vi "Live Capture Functional Stack.10.64bit.vi"() -> ()   [LabVIEW 2014]
uses:
  subvis/Stack Track.ctl
  subvis/Stack_State.ctl
  CameraControlTypeDef.ctl
  Desktop/camtiff/ctiff.llb/__CTIFFNewFileAndStyleUINT16.vi
  Desktop/camtiff/ctiff.llb/__CTIFFAddNewPageUINT16.vi
panel:
  in  "Preview":bool
  in  "Capture Mode":bool
  out "Record Ready":bool
  in  "Stacks":dbl=1.0
  out "Stack Frames":i32=100
  in  "Stack Frames":i32=100
  in  "Temp":path=path "C:/temp.tmp"
  in  "Frames":i32=100
  in  "HardDisk Record":bool
  in  "Internal Line Interval":dbl
  in  "Slit Width / Lines":sgl=150.0
  in  "Camera Readout Mode":u16(ring)=12 items=["Full Frame"=1, "Slit Scanning"=12]
  in  "Readout Direction":sgl(ring)=1.0 items=["Forward"=1, "Backward"=2]
  in  "Trigger Mode":sgl(ring)=1.0 items=["Normal"=1, "Start "=6]
  in  "Trigger Source":sgl(ring)=2.0 items=["Internal"=1, "External"=2]
  out "State":T1=enum."Start Sequence"
  out "Image":u16[][](graph)
  out "Saving":bool
  in  "AutoIncrement":bool=TRUE
  in  "Path":path=path "C:/Users/spim/Desktop/Craig Cap/temp/a.tiff"
  in  "Frames":i32=100
  out "Frame Index":i32
  out "error out":errorcluster
  in  "stop":bool
  in  "Ram Record":bool
  out "Total Frames":i32
  out "Elapsed Time":u32
  out "Software FPS":dbl
  out "Camera FPS":dbl
  in  "H Offset":i32 min=0 max=0 step=4
  in  "H Width":i32 min=4 max=2048 step=4
  out "SMD":dbl
  out "SHO":i32
  in  "V Offset":i32 min=0 max=0 step=4
  in  "V Width":i32 min=4 max=2048 step=4
  in  "Binning":u16(ring) items=["1x1"=1, "2x2"=2, "4x4"=4]
  out "SHW":i32
  out "SVO":i32
  out "SVW":i32
  in  "Scan Mode":dbl min=1.0 max=2.0 step=1.0
  in  "Exposure":dbl min=0.0010036691729323308 max=10.000004210526315 step=1e-08
  out "EXP":dbl
  out "Camera Model":string
  out "Camera Version":string
  out "Camera Serial":string
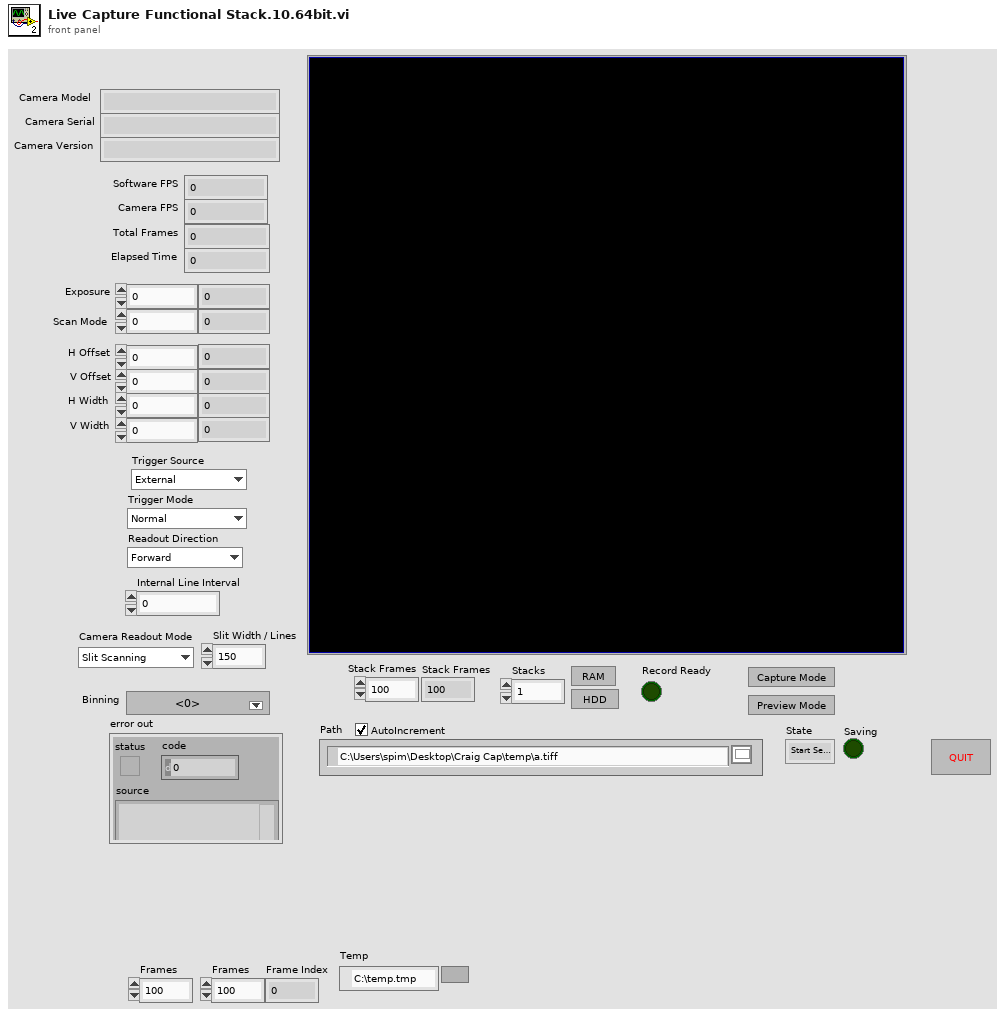
[diagram p1: front panel]
types:
  T1 = typedef "Stack Track.ctl" = enum16{"Idle", "Start Sequence", "Read Disk", "STOP", "Collecting", "End"}
  T2 = typedef "CameraControlTypeDef.ctl" = enum16{"IntervalLineInt", "Ram Record", "HardDisk Record", "Disengage Update", "Update", "Idle", "ROI", "Binning", "Scan Mode", "Trigger Mode", "Readout Mode", "Readout Direction", "Preview"}
  T3 = typedef "Stack_State.ctl" = cluster{"State":T1, "Stack Number":i32, "Image":u16[][], "Stacks":i32}
  T4 = enum8{"Enabled", "Disabled", "Disabled and Grayed Out"}
  T5 = cluster{"Model":string, "Camera ID":string, "Firmware":string}
  T6 = cluster{"Value":i32, "Minimum":i32, "Maximum":i32, "Increment":i32}
  T7 = cluster{"height":u32, "width":u32, "datatype":u32}
  T8 = cluster{"H Offset":i32, "V Offset":i32, "H Width":i32, "V Width":i32}
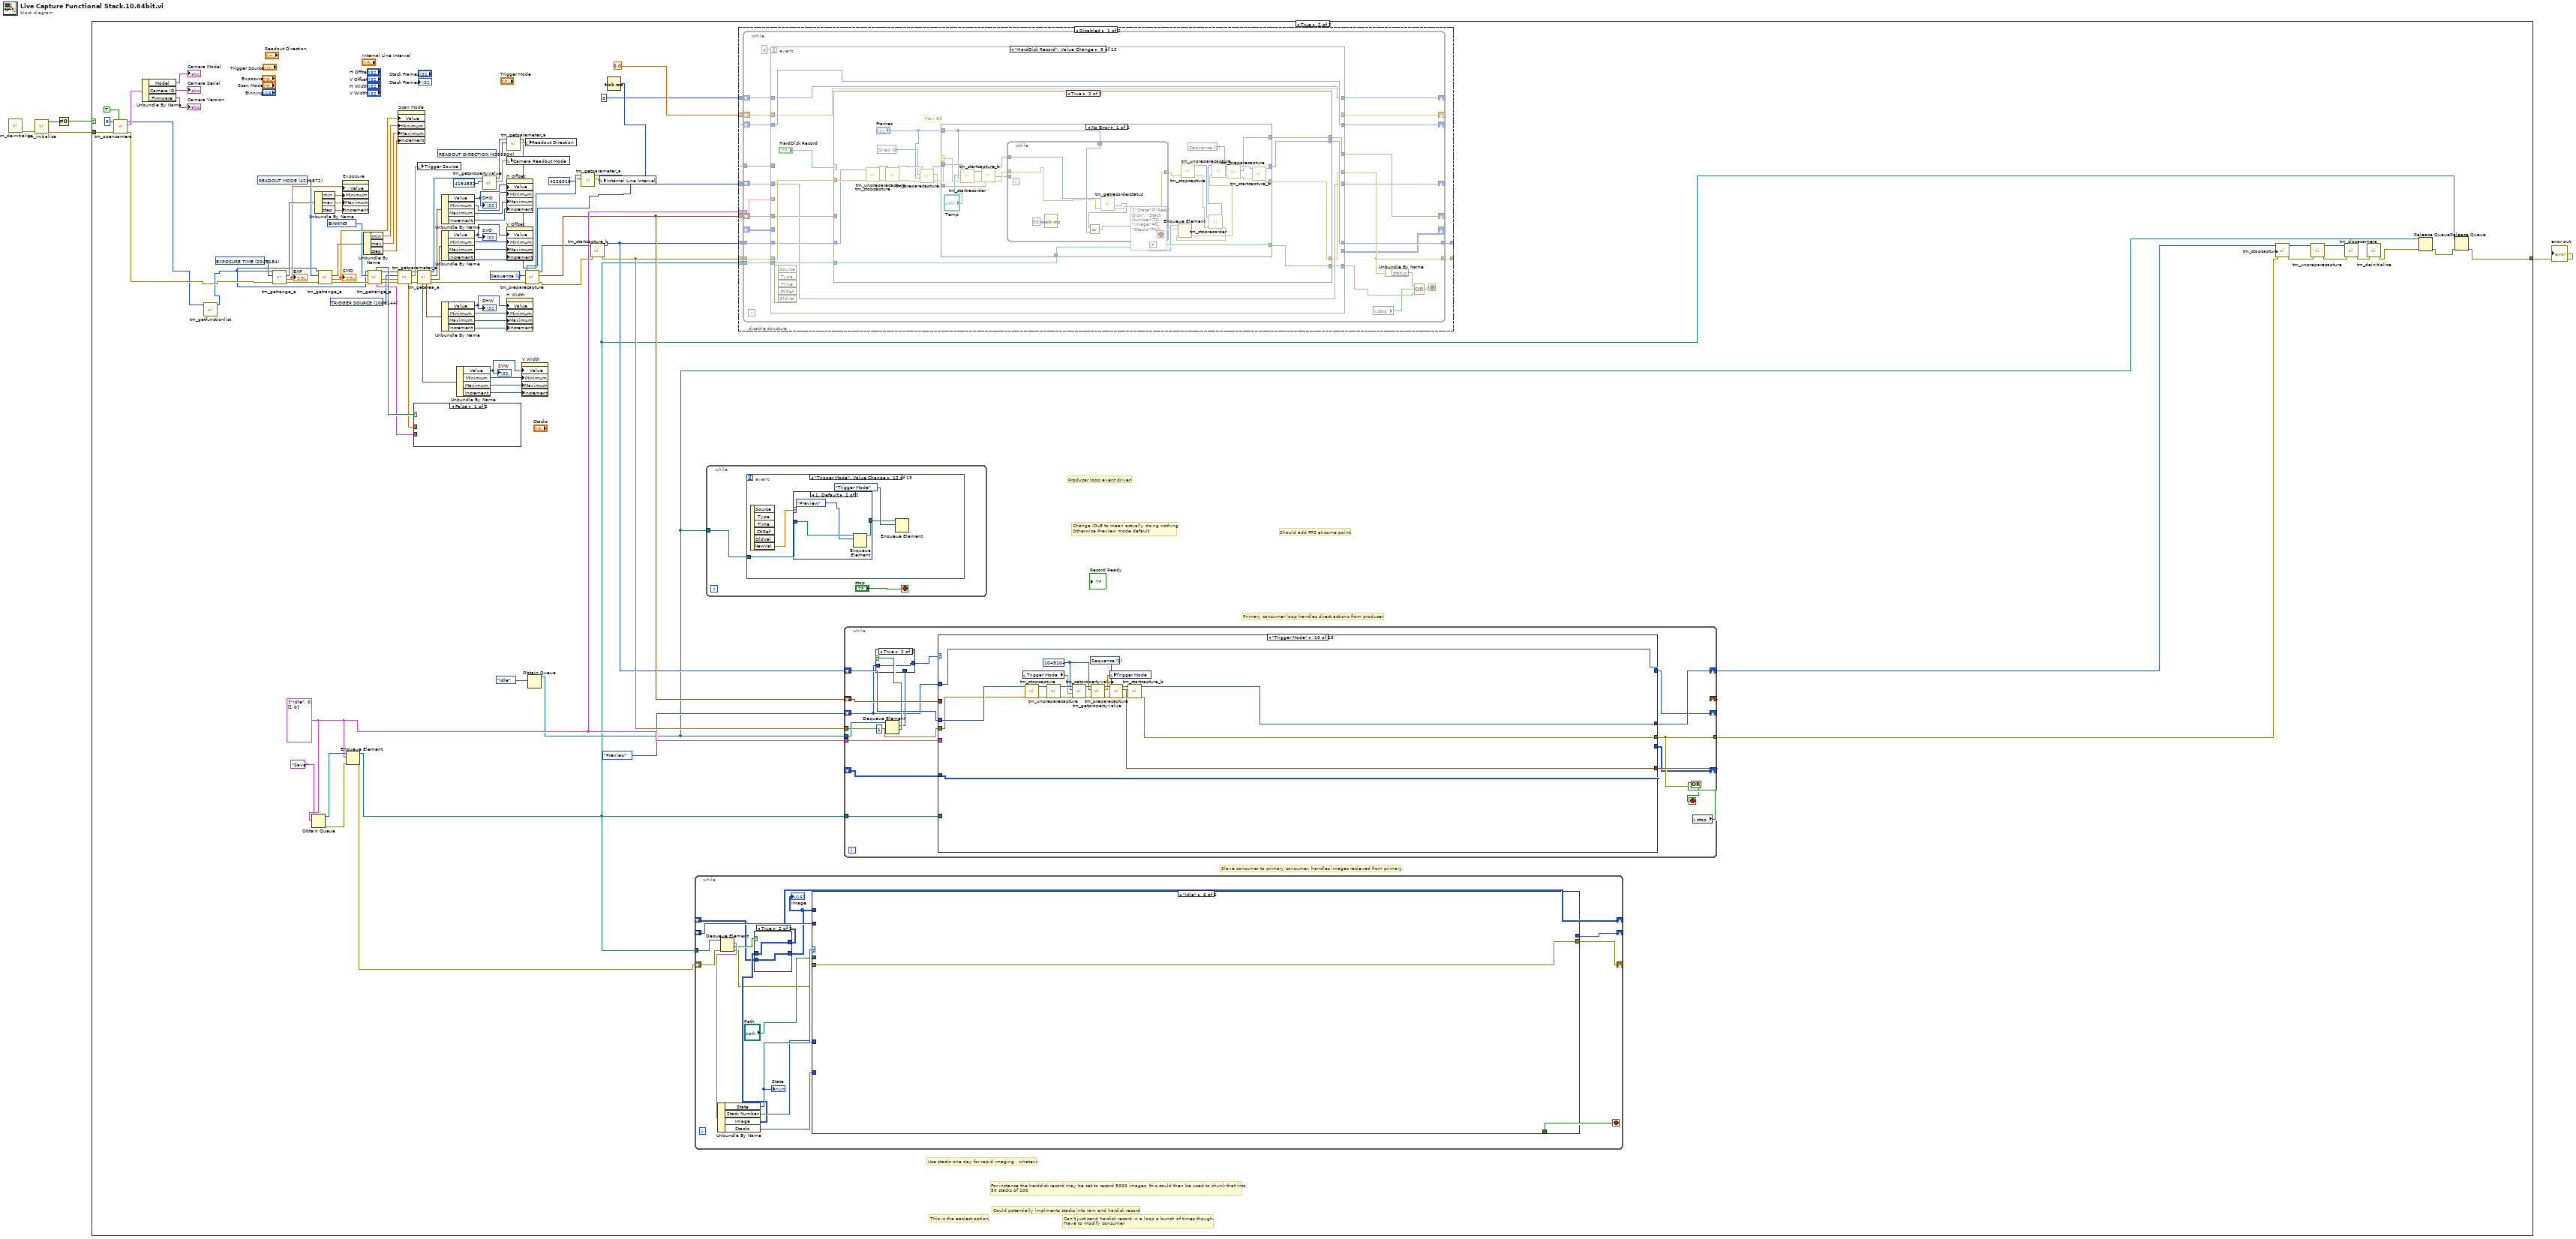
[diagram p0: block diagram]
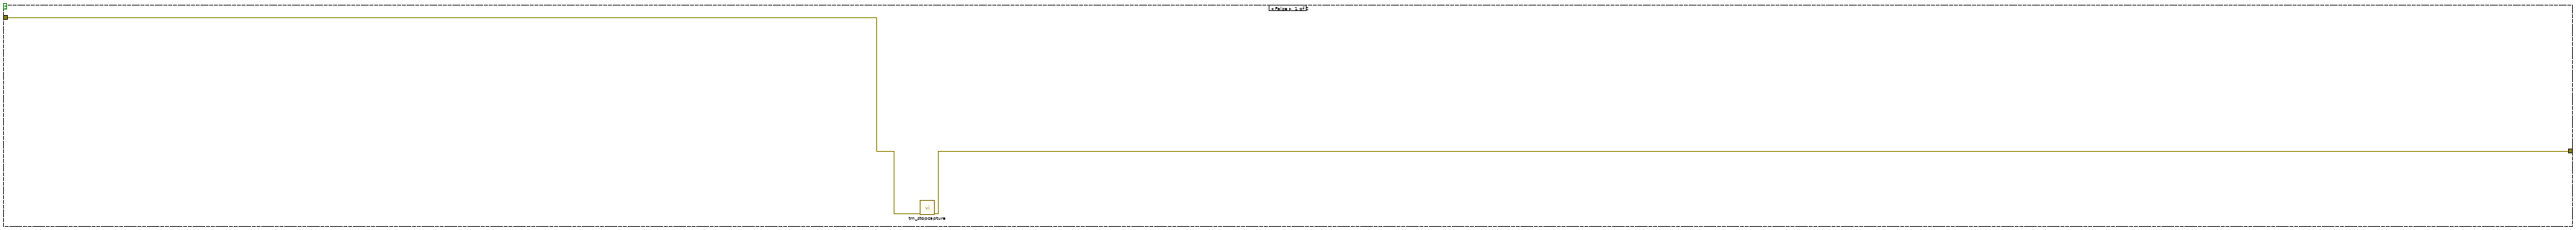
[diagram p2: hidden frame]
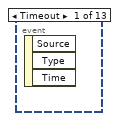
[diagram p3: hidden frame]
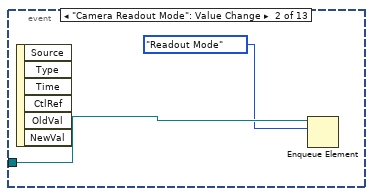
[diagram p4: hidden frame]
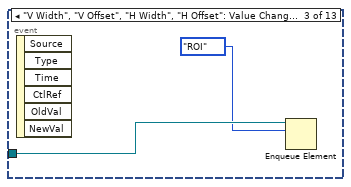
[diagram p5: hidden frame]
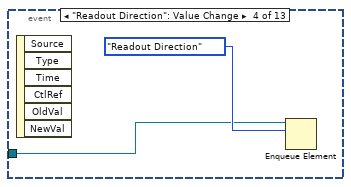
[diagram p6: hidden frame]
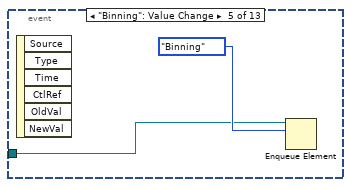
[diagram p7: hidden frame]
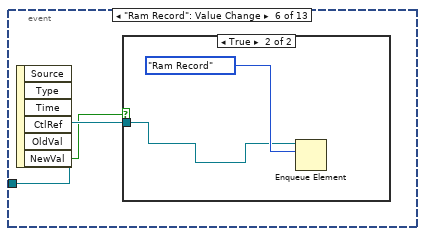
[diagram p8: hidden frame]
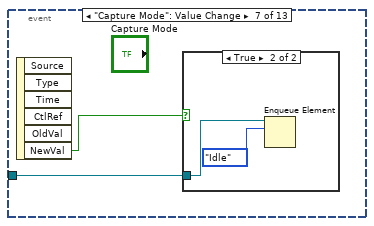
[diagram p10: hidden frame]
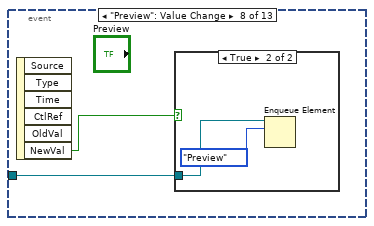
[diagram p12: hidden frame]
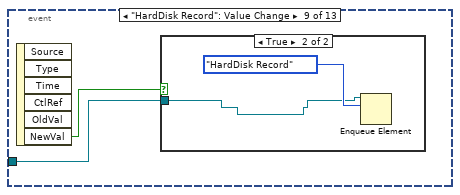
[diagram p14: hidden frame]
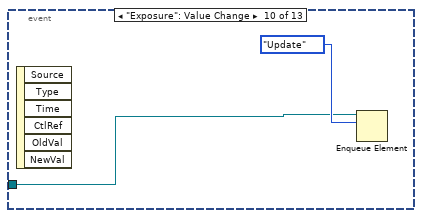
[diagram p16: hidden frame]
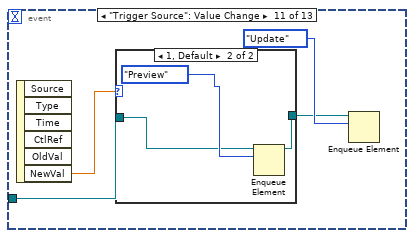
[diagram p17: hidden frame]
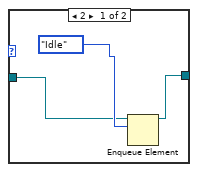
[diagram p18: hidden frame]
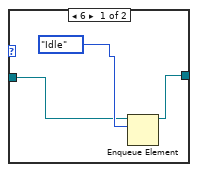
[diagram p19: hidden frame]
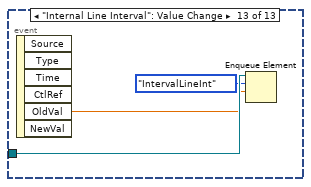
[diagram p20: hidden frame]
diagram:
  n1 = call <userlib>:"tm_deinitialize.vi"() -> ("error out"=w1:errorcluster)  [unwired: 11 in]
  n2 = call <userlib>:"tm_initialize.vi"("error in (no error)"=w1) -> ("error out"=w3:errorcluster, "Number Of Cameras"=w2:u32)  [unwired: 7 in, 2 out]
  n3 = Not Equal To 0?(x=w2) -> (x != 0?=w5:bool)
  n4 = case shown="True" w5 {
    tunnel: [w6 w17] -> w4
    tunnel: w3 -> [w7 w100]
    frame False {
      n5 = call <userlib>:"tm_stopcapture.vi"("error in (no error)"=w7) -> ("error out"=w6:errorcluster)  [unwired: 9 in, 1 out]
    }
    frame True {
      w35 = u32 4211904 items=["SENSOR MODE"=4212128, "CCD MODE"=4212384, "READOUT MODE"=4211872, "ACTIVE VIEW INDEX"=4343136, "BITS PER CHANNEL"=4342976, "IMAGE PIXEL TYPE"=4343296, "BINNING"=4215968, "EXPOSURE TIME"=2049184, "CONTRAST GAIN"=3163312, "CONTRAST OFFSET"=3163328, "LIGHT MODE"=2114720, "SENSITIVITY"=2114992, "PHOTON IMAGING MODE"=2115200, "HIGH DYNAMIC RANGE MODE"=3163360, "WHITE BALANCE"=3163568, "TEMPERATURE"=2115232, "TEMPERATURE TARGET"=2115264, "SENSOR COOLER FAN"=2115296, "LINEBUNDLE HEIGHT"=4212192, "MECHANICAL SHUTTER"=2115488, "BACK FOCUS POSITION"=8422304, "TRIGGER CONNECTOR"=1066432, "TRIGGER SOURCE"=1066144, "OUTPUT TRIGGER SOURCE"=1852576, "TRIGGER GLOBAL EXPOSURE"=2049680, "FIRST TRIGGER BEHAVIOR"=2049696, "CHANNEL SYNC"=1852352, "READOUT DIRECTION"=4211904, "PRE HSYNC COUNT"=1852704] ("Parameter")
      w44 = u32 1066144 items=["SENSOR MODE"=4212128, "CCD MODE"=4212384, "READOUT MODE"=4211872, "ACTIVE VIEW INDEX"=4343136, "BITS PER CHANNEL"=4342976, "IMAGE PIXEL TYPE"=4343296, "BINNING"=4215968, "EXPOSURE TIME"=2049184, "CONTRAST GAIN"=3163312, "CONTRAST OFFSET"=3163328, "LIGHT MODE"=2114720, "SENSITIVITY"=2114992, "PHOTON IMAGING MODE"=2115200, "HIGH DYNAMIC RANGE MODE"=3163360, "WHITE BALANCE"=3163568, "TEMPERATURE"=2115232, "TEMPERATURE TARGET"=2115264, "SENSOR COOLER FAN"=2115296, "LINEBUNDLE HEIGHT"=4212192, "MECHANICAL SHUTTER"=2115488, "BACK FOCUS POSITION"=8422304, "TRIGGER CONNECTOR"=1066432, "TRIGGER SOURCE"=1066144, "OUTPUT TRIGGER SOURCE"=1852576, "TRIGGER GLOBAL EXPOSURE"=2049680, "FIRST TRIGGER BEHAVIOR"=2049696, "CHANNEL SYNC"=1852352, "READOUT DIRECTION"=4211904, "PRE HSYNC COUNT"=1852704] ("Parameter")
      w30 = T3 {"State"=enum."Idle", "Stack Number"=0, "Image"=[], "Stacks"=0} ("input cluster")
      w49 = u32 2049184 items=["BINNING"=4215968, "BITS PER CHANNEL"=4342976, "ACTIVE VIEW INDEX"=4343136, "CCD MODE"=4212384, "SENSOR MODE"=4212128, "READOUT MODE"=4211872, "EXPOSURE TIME"=2049184, "CONTRAST GAIN"=3163312, "CONTRAST OFFSET"=3163328, "LIGHT MODE"=2114720, "SENSITIVITY"=2114992, "WHITE BALANCE"=3163568, "PHOTON IMAGING MODE"=2115200, "HIGH DYNAMIC RANGE MODE"=3163360, "TRIGGER SOURCE"=1066144, "TRIGGER ACTIVE"=1066160, "TRIGGER MODE"=1066400, "TRIGGER POLARITY"=1066416, "TRIGGER GLOBAL EXPOSURE"=2049680, "FIRST TRIGGER BEHAVIOR"=2049696, "TRIGGER TIMES"=1066448, "OUTPUT TRIGGER POLARITY"=1852592, "OUTPUT TRIGGER DELAY"=1852624, "OUTPUT TRIGGER PERIOD"=1852640, "TEMPERATURE"=2115232, "TEMPERATURE TARGET"=2115264, "SENSOR COOLER FAN"=2115296, "MECHANICAL SHUTTER"=2115488, "BACK FOCUS POSITION"=8422304, "FRAMEBUNDLE MODE"=4346784, "FRAMEBUNDLE NUMBER"=4346800, "LINEBUNDLE HEIGHT"=4212192, "TRIGGER CONNECTOR"=1066432, "IMAGE PIXEL TYPE"=4343296, "OUTPUT TRIGGER KIND"=1852656, "READOUT DIRECTION"=4211904, "CHANNEL SYNC"=1852352] ("Parameter")
      w50 = u32 4211872 items=["BINNING"=4215968, "BITS PER CHANNEL"=4342976, "ACTIVE VIEW INDEX"=4343136, "CCD MODE"=4212384, "SENSOR MODE"=4212128, "READOUT MODE"=4211872, "EXPOSURE TIME"=2049184, "CONTRAST GAIN"=3163312, "CONTRAST OFFSET"=3163328, "LIGHT MODE"=2114720, "SENSITIVITY"=2114992, "WHITE BALANCE"=3163568, "PHOTON IMAGING MODE"=2115200, "HIGH DYNAMIC RANGE MODE"=3163360, "TRIGGER SOURCE"=1066144, "TRIGGER ACTIVE"=1066160, "TRIGGER MODE"=1066400, "TRIGGER POLARITY"=1066416, "TRIGGER GLOBAL EXPOSURE"=2049680, "FIRST TRIGGER BEHAVIOR"=2049696, "TRIGGER TIMES"=1066448, "OUTPUT TRIGGER POLARITY"=1852592, "OUTPUT TRIGGER DELAY"=1852624, "OUTPUT TRIGGER PERIOD"=1852640, "TEMPERATURE"=2115232, "TEMPERATURE TARGET"=2115264, "SENSOR COOLER FAN"=2115296, "MECHANICAL SHUTTER"=2115488, "BACK FOCUS POSITION"=8422304, "FRAMEBUNDLE MODE"=4346784, "FRAMEBUNDLE NUMBER"=4346800, "LINEBUNDLE HEIGHT"=4212192, "TRIGGER CONNECTOR"=1066432, "IMAGE PIXEL TYPE"=4343296, "OUTPUT TRIGGER KIND"=1852656, "READOUT DIRECTION"=4211904, "CHANNEL SYNC"=1852352] ("Parameter")
      w51 = u32 4215968 items=["BINNING"=4215968, "BITS PER CHANNEL"=4342976, "ACTIVE VIEW INDEX"=4343136, "CCD MODE"=4212384, "SENSOR MODE"=4212128, "READOUT MODE"=4211872, "EXPOSURE TIME"=2049184, "CONTRAST GAIN"=3163312, "CONTRAST OFFSET"=3163328, "LIGHT MODE"=2114720, "SENSITIVITY"=2114992, "WHITE BALANCE"=3163568, "PHOTON IMAGING MODE"=2115200, "HIGH DYNAMIC RANGE MODE"=3163360, "TRIGGER SOURCE"=1066144, "TRIGGER ACTIVE"=1066160, "TRIGGER MODE"=1066400, "TRIGGER POLARITY"=1066416, "TRIGGER GLOBAL EXPOSURE"=2049680, "FIRST TRIGGER BEHAVIOR"=2049696, "TRIGGER TIMES"=1066448, "OUTPUT TRIGGER POLARITY"=1852592, "OUTPUT TRIGGER DELAY"=1852624, "OUTPUT TRIGGER PERIOD"=1852640, "TEMPERATURE"=2115232, "TEMPERATURE TARGET"=2115264, "SENSOR COOLER FAN"=2115296, "MECHANICAL SHUTTER"=2115488, "BACK FOCUS POSITION"=8422304, "FRAMEBUNDLE MODE"=4346784, "FRAMEBUNDLE NUMBER"=4346800, "LINEBUNDLE HEIGHT"=4212192, "TRIGGER CONNECTOR"=1066432, "IMAGE PIXEL TYPE"=4343296, "OUTPUT TRIGGER KIND"=1852656, "READOUT DIRECTION"=4211904, "CHANNEL SYNC"=1852352] ("Parameter")
      w96 = 1 items=["Snap", "Sequence"] ("Capture mode")
      # "Can't just send hardisk record in a loop a bunch of times though.\nHave to modify consumer"
      # "This is the easiest option."
      # "Could potentially implments stacks into ram and hardisk record"
      # "For instance the harddisk record may be set to record 5000 images, this could then be used to chunk that into\n50 stacks of 100"
      # "Use stacks one day for rapid imaging , whatevr."
      # "Change IDLE to mean actually doing nothing\nOtherwise Preview mode default"
      # "Slave consumer to primary consumer, handles images recieved from primary."
      # "Primary consumer loop handles direct actions from producer"
      # "Producer loop event driven"
      # "Should add FPS at some point."
      n6 = call <userlib>:"tm_opencamera.vi"("Force Open"=TRUE, "error in (no error)"=w100, "Camera Index"=u32 0) -> ("error out"=w31:errorcluster, "Camera Details"=w63:T5, "Handle out"=w15:u32)  [unwired: 6 in]
      n7 = Unbundle By Name(w63) -> ("Model"=→"Camera Model":string, "Camera ID"=→"Camera Serial":string, "Firmware"=→"Camera Version":string)
      n8 = call <userlib>:"tm_getfunctionlist.vi"("Handle in"=w15) -> ("Handle out"=w14:u32)  [unwired: 8 in, 2 out]
      n9 = call <userlib>:"tm_getrange_a.vi"("error in (no error)"=w31, "Parameter"=w49, "Handle in"=w14) -> ("error out"=w58:errorcluster, "default"=w47:dbl, "Range"=w59:cluster{"min":dbl, "max":dbl, "step":dbl})  [unwired: 2 in, 4 out]
      "EXP" <- w47
      n10 = Obtain Queue(name (unnamed)="Save", element data type=w30) -> (queue out=w33:refnum<queue>, error out=w12:errorcluster)  [unwired: 3 in, 1 out]
      n11 = Unbundle By Name(w59) -> ("min"=w94:dbl, "max"=w93:dbl, "step"=w92:dbl)
      n12 = call <userlib>:"tm_getrange_a.vi"("error in (no error)"=w58, "Parameter"=w50, "Handle in"=w14) -> ("error out"=w55:errorcluster, "default"=w56:dbl, "Range"=w57:cluster{"min":dbl, "max":dbl, "step":dbl})  [unwired: 2 in, 4 out]
      "SMD" <- w56
      n13 = property on="Exposure" class="DigNum (strict)"("Value"=w47, "Minimum"=w94, "Maximum"=w93, "Increment"=w92) -> ()  [unwired: 2 in, 2 out]
      n14 = Enqueue Element(queue=w33, element=w30, error in (no error)=w12) -> (queue out=w16:refnum<queue>, error out=w11:errorcluster)  [unwired: 1 in, 1 out]
      n15 = Unbundle By Name(w57) -> ("min"=w91:dbl, "max"=w90:dbl, "step"=w89:dbl)
      n16 = call <userlib>:"tm_getrange_a.vi"("error in (no error)"=w55, "Parameter"=w51, "Handle in"=w14) -> ("error out"=w41:errorcluster, "default"=w53:dbl, "Handle out"=w43:u32, "Value Names"=w52:cluster{"Name":string, "Value":dbl}[], "Writable"=w54:bool)  [unwired: 2 in, 2 out]
      n17 = property on="Scan Mode" class="DigNum (strict)"("Value"=w56, "Minimum"=w91, "Maximum"=w90, "Increment"=w89) -> ()  [unwired: 2 in, 2 out]
      n18 = call <userlib>:"tm_getparameter_a.vi"("error in (no error)"=w41, "Parameter"=w44, "Handle in"=w43) -> ("error out"=w40:errorcluster, "Value out"=w45:dbl, "Handle out"=w42:u32)  [unwired: 6 in]
      n19 = case shown="False" w54 {
        tunnel: w52 -> [_ w1193]
        tunnel: w53 -> [_ w1192]
        frame False {
        }
        frame True {
          n20 = property on="Binning" class="Ring (strict)"("Value"=w1192, "StringsAndValues[]"=w1193) -> ()  [unwired: 2 in, 2 out]
        }
      }
      n21 = local write "Trigger Source"(w45) -> ()
      n22 = call <userlib>:"tm_getarea_a.vi"("error in (no error)"=w40, "Handle in"=w42) -> ("error out"=w46:errorcluster, "V Offset"=w88:T6, "H Offset"=w69:T6, "Handle out"=w37:u32, "H Width"=w87:T6, "V Width"=w86:T6)  [unwired: 4 in]
      n23 = Unbundle By Name(w69) -> ("Value"=w68:i32, "Minimum"=w67:i32, "Maximum"=w66:i32, "Increment"=w65:i32)
      "SHO" <- w68
      n24 = Unbundle By Name(w88) -> ("Value"=w76:i32, "Minimum"=w85:i32, "Maximum"=w84:i32, "Increment"=w83:i32)
      "SVO" <- w76
      n25 = Unbundle By Name(w87) -> ("Value"=w75:i32, "Minimum"=w82:i32, "Maximum"=w81:i32, "Increment"=w80:i32)
      "SHW" <- w75
      n26 = Unbundle By Name(w86) -> ("Value"=w74:i32, "Minimum"=w79:i32, "Maximum"=w78:i32, "Increment"=w77:i32)
      "SVW" <- w74
      n27 = call <userlib>:"tm_getpropertyvalue.vi"("Property ID"=u32 4194832, "Handle in"=w37) -> ("Value in"=w38:sgl, "Handle out"=w36:u32)  [unwired: 7 in, 1 out]
      n28 = call <userlib>:"tm_getparameter_a.vi"("Parameter"=w35, "Handle in"=w36) -> ("Value out"=w34:dbl, "Handle out"=w21:u32)  [unwired: 7 in, 1 out]
      n29 = local write "Camera Readout Mode"(w38) -> ()
      n30 = property on="H Offset" class="DigNum (strict)"("Value"=w68, "Minimum"=w67, "Maximum"=w66, "Increment"=w65) -> ()  [unwired: 2 in, 2 out]
      n31 = property on="V Offset" class="DigNum (strict)"("Value"=w76, "Minimum"=w85, "Maximum"=w84, "Increment"=w83) -> ()  [unwired: 2 in, 2 out]
      n32 = property on="H Width" class="DigNum (strict)"("Value"=w75, "Minimum"=w82, "Maximum"=w81, "Increment"=w80) -> ()  [unwired: 2 in, 2 out]
      n33 = property on="V Width" class="DigNum (strict)"("Value"=w74, "Minimum"=w79, "Maximum"=w78, "Increment"=w77) -> ()  [unwired: 2 in, 2 out]
      n34 = local write "Readout Direction"(w34) -> ()
      n35 = Obtain Queue(element data type=CameraControlTypeDef."Idle" ("Enum")) -> (queue out=w19:refnum<queue>)  [unwired: 4 in, 2 out]
      n36 = call <userlib>:"tm_getparameter_a.vi"("Parameter"=4226016, "Handle in"=w21) -> ("Value out"=w9:dbl, "Handle out"=w10:u32)  [unwired: 7 in, 1 out]
      n37 = call <userlib>:"tm_preparecapture.vi"("error in (no error)"=w46, "Capture mode"=w96, "Handle in"=w10) -> ("error out"=w32:errorcluster, "Buffer Info"=w29:T7, "Handle out"=w22:u32)  [unwired: 5 in, 1 out]
      n38 = call <userlib>:"tm_startcapture_b.vi"("error in (no error)"=w32, "Handle in"=w22) -> ("error out"=w27:errorcluster, "Handle out"=w28:u32)  [unwired: 8 in]
      n39 = local write "Internal Line Interval"(w9) -> ()
      n40 = Tick Count (ms)() -> (millisecond timer value=w95:u32)
      n41 = while {
        tunnel: w16 -> [w1109]
        shift-right: [w1105] -> _
        shift-left: _ -> [w1103]
        shift-right: [w1102] -> _
        shift-left: w11 -> [w1095]
        shift-right: [w1100] -> _
        shift-left: _ -> [w1096]
        stop <- w1104 stop-if-true
        n42 = Dequeue Element(queue=w1109, error in (no error)=w1095) -> (element=w1108:T3, timed out?=w1097:bool, error out=w1094:errorcluster)  [unwired: 1 in, 1 out]
        n43 = Unbundle By Name(w1108) -> ("State"=w1107:T1, "Stack Number"=w1106:i32, "Image"=w1098:u16[][], "Stacks"=w1093:i32)
        "State" <- w1107
        n44 = case shown="True" w1097 {
          tunnel: w1098 -> [w1111 w1113]
          tunnel: [w1111 w1112] -> w1099
          tunnel: [w1110 w1113] -> w1100
          tunnel: w1096 -> [w1110 w1112]
          frame False {
          }
          frame True {
          }
        }
        "Image" <- w1099
        n45 = case shown="\"Idle\"" w1107 {
          tunnel: w1106 -> [_ _ _ _ _ _]
          tunnel: [w1116 w1133 _ _ _ _] -> w1105
          tunnel: w1103 -> [_ w1134 w1140 _ _ _]
          tunnel: [FALSE _ _ _ TRUE _] -> w1104
          tunnel: w1099 -> [w1114 w1135 _ _ _ _]
          tunnel: w1094 -> [_ w1132 w1138 w1153 w1189 w1191]
          tunnel: [w1117 w1131 w1139 w1150 w1189 w1191] -> w1102
          tunnel: "Path" -> [w1120 _ _ w1143 _ _]
          tunnel: w1093 -> [_ _ _ w1146 _ _]
          frame "Start Sequence" {
            # "Public tiff library"
            # "Get path and open file"
            n46 = Equal?(x=w1120, y=path "") -> (x = y?=w1122:bool)
            n47 = case shown="True" w1122 {
              tunnel: w1120 -> [w1124 _]
              tunnel: [w1124 w1127] -> w1119
              frame False {
              }
              frame True {
                n48 = call "File Dialog"("pattern (all files)"=".tiff", "pattern label"="Tiff Image") -> ("selected path"=w1127:path)  [unwired: 10 in, 3 out]
              }
            }
            n49 = case shown="True" "AutoIncrement" {
              tunnel: w1119 -> [w1128 w1130]
              tunnel: [w1128 w1129] -> w1115
              frame False {
              }
              frame True {
                n50 = call "4Digit File Incrementer.vi"("path"=w1130) -> ("appended path"=w1129:path)  [unwired: 10 in]
              }
            }
            n51 = local write "Path"(w1115) -> ()
            n52 = call-poly "CTIFFNewFileAndStyle.vi"("image"=w1114, "output_file"=w1115) -> ("error"=w1117:errorcluster, "CTIFF"=w1116:i64)  [unwired: 8 in]
          }
          frame "Collecting" {
            # "Add Image to write scan line"
            n53 = call-poly "CTIFFAddNewPage.vi"("error"=w1132, "image"=w1135, "CTIFF"=w1134) -> ("error"=w1131:errorcluster, "CTIFF"=w1133:i64)  [unwired: 7 in]
            n54 = property on="Ram Record" class="Bool (strict)"("DisabledEnum"=T4."Disabled and Grayed Out" ("Disabled"), "BoolText.Text"="Saving" ("Boolean Text.Text")) -> ()  [unwired: 2 in, 2 out]
          }
          frame "End" {
            (unwired) FALSE
            # "Close image file, reset capturing button"
            n55 = call "CTIFFWriteAndClose.vi"("error"=w1138, "CTIFF"=w1140) -> ("error"=w1139:errorcluster)  [unwired: 9 in]
            n56 = property on="Ram Record" class="Bool (strict)"("BoolText.Text"="RAM" ("Boolean Text.Text"), "DisabledEnum"=T4."Enabled" ("Disabled")) -> ()  [unwired: 2 in, 2 out]
          }
          frame "Read Disk" {
            n57 = call "4Digit File Incrementer tmp.vi"("Number"=w1146, "path"=path "C:/temp" ("Temp 2")) -> ("appended path"=w1144:path)  [unwired: 9 in]
            n58 = call <userlib>:"tm_opendcimgfile.vi"("Path"=w1144) -> ("Total Frames"=w1155:i32, "File Handle"=w1156:u32)  [unwired: 8 in, 1 out]
            n59 = for {
              N: w1155 -> [_]
              shift-right: [w1163] -> w1151
              shift-left: i64 0 ("CTIFF") -> [w1164]
              tunnel: [w1162] -> w1152
              tunnel: w1153 -> [w1161]
              shift-right: [w1166] -> w1147
              shift-left: w1156 -> [w1167]
              tunnel: w1143 -> [w1157]
              i -> [w1158]
              n60 = local write "Stack Frames"(w1158) -> ()
              n61 = Equal To 0?(x=w1158) -> (x = 0?=w1165:bool)
              n62 = call <userlib>:"tm_getdcimgframe.vi"("error in (no error)"=w1161, "Frame Index"=w1158, "File Handle in"=w1167) -> ("error out"=w1160:errorcluster, "Data"=w1159:u16[][], "File Handle out"=w1166:u32)  [unwired: 5 in, 1 out]
              n63 = local write "Image"(w1159) -> ()
              n64 = case shown="True" w1165 {
                tunnel: w1159 -> [w1168 w1181]
                tunnel: w1164 -> [w1172 _]
                tunnel: [w1171 w1180] -> w1163
                tunnel: [w1170 w1179] -> w1162
                tunnel: w1160 -> [w1169 _]
                tunnel: w1157 -> [_ w1174]
                frame False {
                  n65 = call-poly "CTIFFAddNewPage.vi"("error"=w1169, "image"=w1168, "CTIFF"=w1172) -> ("error"=w1170:errorcluster, "CTIFF"=w1171:i64)  [unwired: 7 in]
                }
                frame True {
                  n66 = Equal?(x=w1174, y=path "") -> (x = y?=w1175:bool)
                  n67 = case shown="False" w1175 {
                    tunnel: [w1182 w1183] -> w1178
                    tunnel: w1174 -> [w1182 _]
                    frame False {
                    }
                    frame True {
                      n68 = call "File Dialog2"("pattern (all files)"=".tiff", "pattern label"="Tiff Image") -> ("selected path"=w1183:path)  [unwired: 10 in, 3 out]
                    }
                  }
                  n69 = local read "AutoIncrement"() -> (w1177:bool)
                  n70 = case shown="False" w1177 {
                    tunnel: w1178 -> [w1186 w1187]
                    tunnel: [w1186 w1188] -> w1173
                    frame False {
                    }
                    frame True {
                      n71 = call "4Digit File Incrementer.vi"("path"=w1187) -> ("appended path"=w1188:path)  [unwired: 10 in]
                    }
                  }
                  n72 = call-poly "CTIFFNewFileAndStyle.vi"("image"=w1181, "output_file"=w1173) -> ("error"=w1179:errorcluster, "CTIFF"=w1180:i64)  [unwired: 8 in]
                  n73 = local write "Path"(w1173) -> ()
                }
              }
            }
            n74 = call "CTIFFWriteAndClose.vi"("error"=w1152, "CTIFF"=w1151) -> ("error"=w1149:errorcluster)  [unwired: 9 in]
            n75 = call <userlib>:"tm_closedcimgfile.vi"("error in (no error)"=w1149, "File Handle"=w1147) -> ("error out"=w1148:errorcluster)  [unwired: 9 in]
            n76 = Delete(path (use dialog)=w1144, error in=w1148) -> (error out=w1150:errorcluster)  [unwired: 3 in, 2 out]
          }
          frame "STOP" {
          }
          frame "Idle" {
          }
        }
      }
      n77 = while {
        tunnel: w19 -> [w102]
        stop <- "stop" stop-if-true
        n78 = event shown="[11] \"Trigger Mode\": Value Change" {
          selector: _ -> [_ _ _ _ _ _ _ _ _ _ _ _ _]
          dyn-events: _ -> [_ _ _ _ _ _ _ _ _ _ _ _ _]
          timeout: _ -> [_ _ _ _ _ _ _ _ _ _ _ _ _]
          tunnel: w102 -> [_ w104 w106 w107 w109 w112 w115 w119 w124 w127 w131 w141 w151]
          event Timeout {
            n79 = event-data() -> ()  [unwired: 1 in, 3 out]
          }
          event "Camera Readout Mode": Value Change {
            n80 = event-data() -> ()  [unwired: 1 in, 6 out]
            n81 = Enqueue Element(queue=w104, element=CameraControlTypeDef."Readout Mode" ("Enum")) -> ()  [unwired: 2 in, 3 out]
          }
          event "V Width", "V Offset", "H Width", "H Offset": Value Change {
            n82 = event-data() -> ()  [unwired: 1 in, 6 out]
            n83 = Enqueue Element(queue=w106, element=CameraControlTypeDef."ROI" ("Enum")) -> ()  [unwired: 2 in, 3 out]
          }
          event "Readout Direction": Value Change {
            n84 = event-data() -> ()  [unwired: 1 in, 6 out]
            n85 = Enqueue Element(queue=w107, element=CameraControlTypeDef."Readout Direction" ("Enum")) -> ()  [unwired: 2 in, 3 out]
          }
          event "Binning": Value Change {
            n86 = event-data() -> ()  [unwired: 1 in, 6 out]
            n87 = Enqueue Element(queue=w109, element=CameraControlTypeDef."Binning" ("Enum")) -> ()  [unwired: 2 in, 3 out]
          }
          event "Ram Record": Value Change {
            n88 = event-data() -> ("NewVal"=w111:bool)  [unwired: 1 in, 5 out]
            n89 = case shown="True" w111 {
              tunnel: w112 -> [_ w113]
              frame False {
              }
              frame True {
                n90 = Enqueue Element(queue=w113, element=CameraControlTypeDef."Ram Record" ("Enum")) -> ()  [unwired: 2 in, 3 out]
              }
            }
          }
          event "Capture Mode": Value Change {
            n91 = event-data() -> ("NewVal"=w116:bool)  [unwired: 1 in, 5 out]
            n92 = case shown="True" w116 {
              tunnel: w115 -> [_ w118]
              frame False {
              }
              frame True {
                n93 = Enqueue Element(queue=w118, element=CameraControlTypeDef."Idle") -> ()  [unwired: 2 in, 3 out]
              }
            }
          }
          event "Preview": Value Change {
            n94 = event-data() -> ("NewVal"=w120:bool)  [unwired: 1 in, 5 out]
            n95 = case shown="True" w120 {
              tunnel: w119 -> [_ w122]
              frame False {
              }
              frame True {
                n96 = Enqueue Element(queue=w122, element=CameraControlTypeDef."Preview") -> ()  [unwired: 2 in, 3 out]
              }
            }
          }
          event "HardDisk Record": Value Change {
            n97 = event-data() -> ("NewVal"=w123:bool)  [unwired: 1 in, 5 out]
            n98 = case shown="True" w123 {
              tunnel: w124 -> [_ w125]
              frame False {
              }
              frame True {
                n99 = Enqueue Element(queue=w125, element=CameraControlTypeDef."HardDisk Record" ("Enum")) -> ()  [unwired: 2 in, 3 out]
              }
            }
          }
          event "Exposure": Value Change {
            n100 = event-data() -> ()  [unwired: 1 in, 6 out]
            n101 = Enqueue Element(queue=w127, element=CameraControlTypeDef."Update" ("Enum")) -> ()  [unwired: 2 in, 3 out]
          }
          event "Trigger Source": Value Change {
            n102 = event-data() -> ("NewVal"=w129:sgl)  [unwired: 1 in, 5 out]
            n103 = case shown="1, Default" w129 {
              tunnel: w131 -> [w134 w137]
              tunnel: [w133 w136] -> w130
              frame 2 {
                n104 = Enqueue Element(queue=w134, element=CameraControlTypeDef."Idle" ("Enum")) -> (queue out=w133:refnum<queue>)  [unwired: 2 in, 2 out]
              }
              frame 1, Default {
                n105 = Enqueue Element(queue=w137, element=CameraControlTypeDef."Preview" ("Enum")) -> (queue out=w136:refnum<queue>)  [unwired: 2 in, 2 out]
              }
            }
            n106 = Enqueue Element(queue=w130, element=CameraControlTypeDef."Update" ("Enum")) -> ()  [unwired: 2 in, 3 out]
          }
          event "Trigger Mode": Value Change {
            n107 = event-data() -> ("NewVal"=w139:sgl)  [unwired: 1 in, 5 out]
            n108 = case shown="1, Default" w139 {
              tunnel: w141 -> [w144 w147]
              tunnel: [w143 w146] -> w140
              frame 6 {
                n109 = Enqueue Element(queue=w144, element=CameraControlTypeDef."Idle" ("Enum")) -> (queue out=w143:refnum<queue>)  [unwired: 2 in, 2 out]
              }
              frame 1, Default {
                n110 = Enqueue Element(queue=w147, element=CameraControlTypeDef."Preview" ("Enum")) -> (queue out=w146:refnum<queue>)  [unwired: 2 in, 2 out]
              }
            }
            n111 = Enqueue Element(queue=w140, element=CameraControlTypeDef."Trigger Mode" ("Enum")) -> ()  [unwired: 2 in, 3 out]
          }
          event "Internal Line Interval": Value Change {
            n112 = event-data() -> ("OldVal"=w150:dbl)  [unwired: 1 in, 5 out]
            n113 = Enqueue Element(queue=w151, element=CameraControlTypeDef."IntervalLineInt", timeout in ms (-1)=w150) -> ()  [unwired: 1 in, 3 out]
          }
        }
      }
      n114 = disable-structure shown="Disabled" {
        disable-tunnel: 0.0 -> [w593 _]
        disable-tunnel: w95 -> [w592 _]
        disable-tunnel: 0 -> [w591 _]
        disable-tunnel: [w590 _] -> _
        disable-tunnel: [w589 _] -> _
        disable-tunnel: w30 -> [w588 _]
        disable-tunnel: w29 -> [w587 _]
        disable-tunnel: w28 -> [w586 _]
        disable-tunnel: w27 -> [w585 _]
        disable-tunnel: w16 -> [w584 _]
        frame Disabled {
          n115 = while {
            tunnel: w585 -> [w607]
            tunnel: [w605] -> w589
            tunnel: [w604] -> w590
            shift-right: [w614] -> _
            shift-left: w592 -> [w612]
            shift-right: [w615] -> _
            shift-left: w593 -> [w613]
            shift-right: [w606] -> _
            shift-left: w592 -> [w610]
            tunnel: w586 -> [w608]
            tunnel: w592 -> [w611]
            shift-right: [w603] -> _
            shift-left: w587 -> [w609]
            shift-right: [w601] -> _
            shift-left: w591 -> [w602]
            tunnel: w584 -> [w600]
            shift-right: [w598] -> _
            shift-left: _ -> [w597]
            tunnel: w588 -> [w596]
            stop <- w616 stop-if-true
            n116 = event shown="[8] \"HardDisk Record\": Value Change" {
              selector: _ -> [_ _ _ _ _ _ _ _ _ _ _ _]
              dyn-events: _ -> [_ _ _ _ _ _ _ _ _ _ _ _]
              timeout: 0 -> [_ _ _ _ _ _ _ _ _ _ _ _]
              tunnel: [w627 w696 w710 w723 w742 w762 w784 w812 w909 w1003 w1039 w1084] -> w615
              tunnel: [w626 w697 w711 w724 w743 w763 w785 w813 w910 w1004 w1040 w1085] -> w614
              tunnel: w613 -> [w638 w696 w710 w723 w742 w762 w784 w812 w909 w1003 w1039 w1084]
              tunnel: w612 -> [w629 w697 w711 w724 w743 w763 w785 w813 w910 w1004 w1040 w1085]
              tunnel: w611 -> [w634 _ _ _ _ _ _ _ _ _ _ _]
              tunnel: w610 -> [w639 w698 w712 w725 w744 w764 w786 w808 w905 w1005 w1047 w1092]
              tunnel: w609 -> [w633 w695 w709 w722 _ w761 _ w809 w906 _ _ _]
              tunnel: w608 -> [w641 w691 w704 w718 w737 w755 w777 w816 w913 w1000 w1016 w1054]
              tunnel: w607 -> [w640 w693 w700 w719 w736 w758 w776 w817 w914 w999 w1015 w1053]
              tunnel: [w637 w698 w712 w725 w744 w764 w786 w808 w905 w1005 w1047 w1092] -> w606
              tunnel: [w636 w688 w707 w715 w728 w748 w767 w814 w911 w994 w1042 w1087] -> w605
              tunnel: [w635 w687 w706 w714 w727 w747 w765 w815 w912 w995 w1043 w1088] -> w604
              tunnel: [w632 w695 w709 w722 w731 w761 w772 w810 w907 w993 w1041 w1086] -> w603
              tunnel: w602 -> [w624 w694 w708 w721 w741 w760 w783 w811 w908 w992 w1012 w1048]
              tunnel: [w623 w694 w708 w721 w741 w760 w783 w811 w908 w992 w1012 w1048] -> w601
              tunnel: w600 -> [w618 _ _ _ _ _ _ w807 w904 _ _ _]
              tunnel: [_ _ _ _ _ _ _ w806 w903 _ _ _] -> w599
              tunnel: w596 -> [w621 _ _ _ _ _ _ w804 _ _ _ _]
              tunnel: [w620 _ _ _ _ _ _ _ _ _ _ _] -> w598
              tunnel: w597 -> [w619 _ _ _ _ _ _ w805 _ _ _ _]
              event Timeout {
                n117 = event-data() -> ()  [unwired: 1 in, 2 out]
                n118 = call <userlib>:"tm_waitnextframe.vi"("error in (no error)"=w640, "Handle in"=w641) -> ("error out"=w644:errorcluster, "Frame Count"=w625:i32, "Frame Index"=w643:i32, "Handle out"=w645:u32)  [unwired: 6 in]
                "Total Frames" <- w625
                n119 = Tick Count (ms)() -> (millisecond timer value=w631:u32)
                n120 = Increment(x=w638) -> (x+1=w628:dbl)
                n121 = Subtract(x=w631, y=w634) -> (x-y=→"Elapsed Time":u32)
                n122 = Add(x=w629, y=u32 1000) -> (x+y=w649:u32)
                n123 = Less Or Equal?(x=w649, y=w631) -> (x <= y?=w630:bool)
                n124 = Add(x=w639, y=u32 50) -> (x+y=w647:u32)
                n125 = Less Or Equal?(x=w647, y=w631) -> (x <= y?=w622:bool)
                n126 = case shown="True" w630 {
                  tunnel: w629 -> [w652 w661]
                  tunnel: [w652 w658] -> w626
                  tunnel: w628 -> [w651 w664]
                  tunnel: w631 -> [_ w658]
                  tunnel: [w651 0.0] -> w627
                  tunnel: w625 -> [_ w653]
                  tunnel: w624 -> [w650 w656]
                  tunnel: [w650 w653] -> w623
                  frame False {
                  }
                  frame True {
                    n127 = Subtract(x=w658, y=w661) -> (x-y=w660:u32)
                    n128 = Subtract(x=w653, y=w656) -> (x-y=w654:i32)
                    n129 = To Double Precision Float(number=w660) -> (double precision float=w666:dbl)
                    n130 = Divide(x=w666, y=1000.0) -> (x/y=w657:dbl)
                    n131 = To Double Precision Float(number=w654) -> (double precision float=w655:dbl)
                    n132 = Divide(x=w655, y=w657) -> (x/y=→"Camera FPS":dbl)
                    n133 = Divide(x=w664, y=w657) -> (x/y=→"Software FPS":dbl)
                  }
                }
                n134 = case shown="True" w622 {
                  tunnel: w639 -> [w671 _]
                  tunnel: w631 -> [_ w684]
                  tunnel: [w671 w684] -> w637
                  tunnel: w645 -> [w670 w683]
                  tunnel: w633 -> [w668 w678]
                  tunnel: w644 -> [w669 w682]
                  tunnel: [w670 w681] -> w636
                  tunnel: [w669 w680] -> w635
                  tunnel: w643 -> [_ w679]
                  tunnel: [w668 w678] -> w632
                  tunnel: w618 -> [_ w677]
                  tunnel: w621 -> [_ w673]
                  tunnel: [w667 w672] -> w620
                  tunnel: w619 -> [w667 _]
                  frame False {
                  }
                  frame True {
                    n135 = call <userlib>:"tm_getframe_a.vi"("error in (no error)"=w682, "Frame Index"=w679, "Buffer Info"=w678, "Handle in"=w683) -> ("error out"=w680:errorcluster, "Data 16"=w672:u16[][], "Handle out"=w681:u32)  [unwired: 3 in, 2 out]
                    n136 = Bundle By Name(cluster=w673, "State"=Stack_Track."Idle", "Stack Number"=0, "Image"=w672) -> (w674:T3)
                    n137 = Enqueue Element(queue=w677, element=w674) -> ()  [unwired: 2 in, 3 out]
                  }
                }
              }
              event "Exposure": Value Change {
                w686 = u32 2049184 items=["SENSOR MODE"=4212128, "CCD MODE"=4212384, "READOUT MODE"=4211872, "ACTIVE VIEW INDEX"=4343136, "BITS PER CHANNEL"=4342976, "IMAGE PIXEL TYPE"=4343296, "BINNING"=4215968, "EXPOSURE TIME"=2049184, "CONTRAST GAIN"=3163312, "CONTRAST OFFSET"=3163328, "LIGHT MODE"=2114720, "SENSITIVITY"=2114992, "PHOTON IMAGING MODE"=2115200, "HIGH DYNAMIC RANGE MODE"=3163360, "WHITE BALANCE"=3163568, "TEMPERATURE"=2115232, "TEMPERATURE TARGET"=2115264, "SENSOR COOLER FAN"=2115296, "LINEBUNDLE HEIGHT"=4212192, "MECHANICAL SHUTTER"=2115488, "BACK FOCUS POSITION"=8422304, "TRIGGER CONNECTOR"=1066432, "TRIGGER SOURCE"=1066144, "OUTPUT TRIGGER SOURCE"=1852576, "TRIGGER GLOBAL EXPOSURE"=2049680, "FIRST TRIGGER BEHAVIOR"=2049696, "CHANNEL SYNC"=1852352, "READOUT DIRECTION"=4211904, "PRE HSYNC COUNT"=1852704] ("Parameter")
                n138 = event-data() -> ("NewVal"=w692:dbl)  [unwired: 1 in, 2 out]
                n139 = call <userlib>:"tm_setparameter_a.vi"("error in (no error)"=w693, "Value in"=w692, "Parameter"=w686, "Handle in"=w691) -> ("error out"=w690:errorcluster, "Handle out"=w689:u32)  [unwired: 6 in]
                n140 = call <userlib>:"tm_getparameter_a.vi"("error in (no error)"=w690, "Parameter"=w686, "Handle in"=w689) -> ("error out"=w687:errorcluster, "Value out"=w685:dbl, "Handle out"=w688:u32)  [unwired: 6 in]
                n141 = local write "EXP"(w685) -> ()
              }
              event "Internal Line Interval": Value Change {
                w699 = u32 4191424 items=["SENSOR MODE"=4212128, "CCD MODE"=4212384, "READOUT MODE"=4211872, "ACTIVE VIEW INDEX"=4343136, "BITS PER CHANNEL"=4342976, "IMAGE PIXEL TYPE"=4343296, "BINNING"=4215968, "EXPOSURE TIME"=2049184, "CONTRAST GAIN"=3163312, "CONTRAST OFFSET"=3163328, "LIGHT MODE"=2114720, "SENSITIVITY"=2114992, "PHOTON IMAGING MODE"=2115200, "HIGH DYNAMIC RANGE MODE"=3163360, "WHITE BALANCE"=3163568, "TEMPERATURE"=2115232, "TEMPERATURE TARGET"=2115264, "SENSOR COOLER FAN"=2115296, "LINEBUNDLE HEIGHT"=4212192, "MECHANICAL SHUTTER"=2115488, "BACK FOCUS POSITION"=8422304, "TRIGGER CONNECTOR"=1066432, "TRIGGER SOURCE"=1066144, "OUTPUT TRIGGER SOURCE"=1852576, "TRIGGER GLOBAL EXPOSURE"=2049680, "FIRST TRIGGER BEHAVIOR"=2049696, "CHANNEL SYNC"=1852352, "READOUT DIRECTION"=4211904, "PRE HSYNC COUNT"=1852704, "INTERNAL LINE SPEED"=4191408, "INTERNAL LINE INVERVAL"=4191424] ("Parameter")
                n142 = event-data() -> ("NewVal"=w703:dbl)  [unwired: 1 in, 2 out]
                n143 = call <userlib>:"tm_setparameter_a.vi"("error in (no error)"=w700, "Value in"=w703, "Parameter"=w699, "Handle in"=w704) -> ("error out"=w701:errorcluster, "Handle out"=w702:u32)  [unwired: 6 in]
                n144 = call <userlib>:"tm_getparameter_a.vi"("error in (no error)"=w701, "Parameter"=w699, "Handle in"=w702) -> ("error out"=w706:errorcluster, "Value out"=w705:dbl, "Handle out"=w707:u32)  [unwired: 6 in]
                n145 = local write "Internal Line Interval"(w705) -> ()
              }
              event "Trigger Source": Value Change {
                w720 = u32 1066144 items=["SENSOR MODE"=4212128, "CCD MODE"=4212384, "READOUT MODE"=4211872, "ACTIVE VIEW INDEX"=4343136, "BITS PER CHANNEL"=4342976, "IMAGE PIXEL TYPE"=4343296, "BINNING"=4215968, "EXPOSURE TIME"=2049184, "CONTRAST GAIN"=3163312, "CONTRAST OFFSET"=3163328, "LIGHT MODE"=2114720, "SENSITIVITY"=2114992, "PHOTON IMAGING MODE"=2115200, "HIGH DYNAMIC RANGE MODE"=3163360, "WHITE BALANCE"=3163568, "TEMPERATURE"=2115232, "TEMPERATURE TARGET"=2115264, "SENSOR COOLER FAN"=2115296, "LINEBUNDLE HEIGHT"=4212192, "MECHANICAL SHUTTER"=2115488, "BACK FOCUS POSITION"=8422304, "TRIGGER CONNECTOR"=1066432, "TRIGGER SOURCE"=1066144, "OUTPUT TRIGGER SOURCE"=1852576, "TRIGGER GLOBAL EXPOSURE"=2049680, "FIRST TRIGGER BEHAVIOR"=2049696, "CHANNEL SYNC"=1852352, "READOUT DIRECTION"=4211904, "PRE HSYNC COUNT"=1852704] ("Parameter")
                n146 = event-data() -> ("NewVal"=w713:sgl)  [unwired: 1 in, 3 out]
                n147 = call <userlib>:"tm_setparameter_a.vi"("error in (no error)"=w719, "Value in"=w713, "Parameter"=w720, "Handle in"=w718) -> ("error out"=w717:errorcluster, "Handle out"=w716:u32)  [unwired: 6 in]
                n148 = call <userlib>:"tm_getparameter_a.vi"("error in (no error)"=w717, "Parameter"=w720, "Handle in"=w716) -> ("error out"=w714:errorcluster, "Handle out"=w715:u32)  [unwired: 6 in, 1 out]
              }
              event "Trigger Mode": Value Change {
                w732 = 1 items=["Snap", "Sequence"] ("Capture mode")
                n149 = event-data() -> ("NewVal"=w726:sgl)  [unwired: 1 in, 4 out]
                n150 = call <userlib>:"tm_stopcapture.vi"("error in (no error)"=w736, "Handle in"=w737) -> ("error out"=w739:errorcluster, "Handle out"=w738:u32)  [unwired: 8 in]
                n151 = call <userlib>:"tm_unpreparecapture.vi"("error in (no error)"=w739, "Handle in"=w738) -> ("error out"=w735:errorcluster, "Handle out"=w734:u32)  [unwired: 8 in]
                n152 = call <userlib>:"tm_setpropertyvalue.vi"("error in (no error)"=w735, "Value in"=w726, "Property ID"=u32 1049104, "Handle in"=w734) -> ("error out"=w730:errorcluster, "Handle out"=w733:u32)  [unwired: 6 in]
                n153 = call <userlib>:"tm_preparecapture.vi"("Capture mode"=w732, "Handle in"=w733) -> ("Buffer Info"=w731:T7, "Handle out"=w729:u32)  [unwired: 6 in, 2 out]
                n154 = call <userlib>:"tm_startcapture_b.vi"("error in (no error)"=w730, "Handle in"=w729) -> ("error out"=w727:errorcluster, "Handle out"=w728:u32)  [unwired: 8 in]
              }
              event "Readout Direction": Value Change {
                w753 = 1 items=["Snap", "Sequence"] ("Capture mode")
                w746 = u32 4211904 items=["SENSOR MODE"=4212128, "CCD MODE"=4212384, "READOUT MODE"=4211872, "ACTIVE VIEW INDEX"=4343136, "BITS PER CHANNEL"=4342976, "IMAGE PIXEL TYPE"=4343296, "BINNING"=4215968, "EXPOSURE TIME"=2049184, "CONTRAST GAIN"=3163312, "CONTRAST OFFSET"=3163328, "LIGHT MODE"=2114720, "SENSITIVITY"=2114992, "PHOTON IMAGING MODE"=2115200, "HIGH DYNAMIC RANGE MODE"=3163360, "WHITE BALANCE"=3163568, "TEMPERATURE"=2115232, "TEMPERATURE TARGET"=2115264, "SENSOR COOLER FAN"=2115296, "LINEBUNDLE HEIGHT"=4212192, "MECHANICAL SHUTTER"=2115488, "BACK FOCUS POSITION"=8422304, "TRIGGER CONNECTOR"=1066432, "TRIGGER SOURCE"=1066144, "OUTPUT TRIGGER SOURCE"=1852576, "TRIGGER GLOBAL EXPOSURE"=2049680, "FIRST TRIGGER BEHAVIOR"=2049696, "CHANNEL SYNC"=1852352, "READOUT DIRECTION"=4211904, "PRE HSYNC COUNT"=1852704] ("Parameter")
                n155 = event-data() -> ("NewVal"=w745:sgl)  [unwired: 1 in, 3 out]
                n156 = call <userlib>:"tm_stopcapture.vi"("error in (no error)"=w758, "Handle in"=w755) -> ("error out"=w759:errorcluster, "Handle out"=w754:u32)  [unwired: 8 in]
                n157 = call <userlib>:"tm_unpreparecapture.vi"("error in (no error)"=w759, "Handle in"=w754) -> ("error out"=w757:errorcluster, "Handle out"=w756:u32)  [unwired: 8 in]
                n158 = call <userlib>:"tm_setparameter_a.vi"("error in (no error)"=w757, "Value in"=w745, "Parameter"=w746, "Handle in"=w756) -> ("error out"=w750:errorcluster, "Handle out"=w749:u32)  [unwired: 6 in]
                n159 = call <userlib>:"tm_preparecapture.vi"("error in (no error)"=w750, "Capture mode"=w753, "Handle in"=w749) -> ("error out"=w751:errorcluster, "Handle out"=w752:u32)  [unwired: 5 in, 2 out]
                n160 = call <userlib>:"tm_startcapture_b.vi"("error in (no error)"=w751, "Handle in"=w752) -> ("error out"=w747:errorcluster, "Handle out"=w748:u32)  [unwired: 8 in]
              }
              event "Camera Readout Mode", "Slit Width / Lines": Value Change {
                w770 = 1 items=["Snap", "Sequence"] ("Capture mode")
                n161 = event-data() -> ()  [unwired: 1 in, 4 out]
                n162 = call <userlib>:"tm_stopcapture.vi"("error in (no error)"=w776, "Handle in"=w777) -> ("error out"=w778:errorcluster, "Handle out"=w774:u32)  [unwired: 8 in]
                n163 = call <userlib>:"tm_unpreparecapture.vi"("error in (no error)"=w778, "Handle in"=w774) -> ("error out"=w769:errorcluster, "Handle out"=w775:u32)  [unwired: 8 in]
                n164 = call <userlib>:"tm_setpropertyvalue.vi"("error in (no error)"=w769, "Value in"="Camera Readout Mode", "Property ID"=u32 4194832, "Handle in"=w775) -> ("error out"=w779:errorcluster, "Handle out"=w780:u32)  [unwired: 6 in]
                n165 = case shown="12" "Camera Readout Mode" {
                  tunnel: w780 -> [w791 w798]
                  tunnel: [w790 w793] -> w773
                  tunnel: w779 -> [w788 w803]
                  tunnel: [w787 w803] -> w771
                  frame 1, Default {
                    n166 = local read "Exposure"() -> (w789:dbl)
                    n167 = call <userlib>:"tm_setpropertyvalue.vi"("error in (no error)"=w788, "Value in"=w789, "Property ID"=u32 2031888, "Handle in"=w791) -> ("error out"=w787:errorcluster, "Handle out"=w790:u32)  [unwired: 6 in]
                  }
                  frame 12 {
                    n168 = local read "Exposure"() -> (w802:dbl)
                    n169 = local read "SVW"() -> (w800:i32)
                    n170 = formula code="slitExpos=frameInter*LW/(LinesToReadout\n+10+LW);\nlineInter = slitExpos / LW;"("frameInter"=w802, "LW"="Slit Width / Lines", "LinesToReadout"=w800) -> ("slitExpos"=w794:dbl, "lineInter"=w797:dbl)
                    n171 = call <userlib>:"tm_setpropertyvalue.vi"("Value in"=w797, "Property ID"=u32 4208720, "Handle in"=w798) -> ("Handle out"=w796:u32)  [unwired: 7 in, 1 out]
                    n172 = call <userlib>:"tm_setpropertyvalue.vi"("Value in"=w794, "Property ID"=u32 2031888, "Handle in"=w796) -> ("Handle out"=w793:u32)  [unwired: 7 in, 1 out]
                  }
                }
                n173 = call <userlib>:"tm_preparecapture.vi"("error in (no error)"=w771, "Capture mode"=w770, "Handle in"=w773) -> ("error out"=w766:errorcluster, "Buffer Info"=w772:T7, "Handle out"=w768:u32)  [unwired: 5 in, 1 out]
                n174 = call <userlib>:"tm_startcapture_b.vi"("error in (no error)"=w766, "Handle in"=w768) -> ("error out"=w765:errorcluster, "Handle out"=w767:u32)  [unwired: 8 in]
              }
              event "Ram Record": Value Change {
                n175 = event-data() -> ()  [unwired: 1 in, 5 out]
                n176 = case shown="True" "Ram Record" {
                  tunnel: w817 -> [w821 w844]
                  tunnel: w816 -> [w820 w841]
                  tunnel: [w821 w827] -> w815
                  tunnel: [w820 w829] -> w814
                  tunnel: [w819 w828] -> w810
                  tunnel: w809 -> [w819 _]
                  tunnel: w807 -> [_ w832]
                  tunnel: [_ w830] -> w806
                  tunnel: w805 -> [_ w826]
                  tunnel: w804 -> [_ w822]
                  frame False {
                  }
                  frame True {
                    w838 = 0 items=["Snap", "Sequence"] ("Capture mode")
                    # "Max 2500"
                    n177 = Flush Queue(queue=w832) -> (queue out=w831:refnum<queue>)  [unwired: 1 in, 2 out]
                    n178 = call <userlib>:"tm_stopcapture.vi"("error in (no error)"=w844, "Handle in"=w841) -> ("error out"=w843:errorcluster, "Handle out"=w842:u32)  [unwired: 8 in]
                    n179 = Bundle By Name(cluster=w822, "State"=Stack_Track."Start Sequence", "Stack Number"=0, "Image"=w826) -> (w823:T3)
                    n180 = call <userlib>:"tm_unpreparecapture.vi"("error in (no error)"=w843, "Handle in"=w842) -> ("error out"=w839:errorcluster, "Handle out"=w840:u32)  [unwired: 8 in]
                    n181 = call <userlib>:"tm_preparecapture.vi"("error in (no error)"=w839, "Frames"="Frames", "Capture mode"=w838, "Handle in"=w840) -> ("error out"=w837:errorcluster, "Buffer Info"=w835:T7, "Handle out"=w836:u32)  [unwired: 4 in, 1 out]
                    n182 = Enqueue Element(queue=w831, element=w823) -> (queue out=w833:refnum<queue>)  [unwired: 2 in, 2 out]
                    n183 = case shown="No Error" w837 {
                      selector: w837 -> [w869 w890]
                      tunnel: w836 -> [w868 w891]
                      tunnel: "Frames" -> [w864 _]
                      tunnel: [w849 w887] -> w829
                      tunnel: w835 -> [w865 _]
                      tunnel: [w848 w889] -> w827
                      tunnel: w833 -> [w863 w885]
                      tunnel: w822 -> [w862 _]
                      tunnel: [w847 w885] -> _
                      tunnel: [FALSE ("value") w899] -> w830
                      tunnel: [w846 w888] -> w828
                      frame No Error {
                        w854 = 1 items=["Snap", "Sequence"] ("Capture mode")
                        # "Frames in RAM"
                        n184 = call <userlib>:"tm_startcapture_b.vi"("error in (no error)"=w869, "Handle in"=w868) -> ("error out"=w866:errorcluster, "Handle out"=w867:u32)  [unwired: 8 in]
                        n185 = for {
                          N: w864 -> [_]
                          tunnel: w867 -> [w884]
                          tunnel: w866 -> [w883]
                          tunnel: w865 -> [w880]
                          tunnel: [w879] -> w860
                          tunnel: [w878] -> w859
                          tunnel: w863 -> [w876]
                          tunnel: Stack_Track."Collecting" ("Enum") -> [w874]
                          tunnel: w862 -> [w872]
                          tunnel: [w871] -> w853
                          i -> [w873]
                          n186 = call <userlib>:"tm_waitnextframe.vi"("error in (no error)"=w883, "Handle in"=w884) -> ("error out"=w881:errorcluster, "Frame Index"=→"Frame Index":i32, "Handle out"=w882:u32)  [unwired: 6 in, 1 out]
                          n187 = call <userlib>:"tm_getframe_a.vi"("error in (no error)"=w881, "Frame Index"=w873, "Buffer Info"=w880, "Handle in"=w882) -> ("error out"=w878:errorcluster, "Data 16"=w870:u16[][], "Handle out"=w879:u32)  [unwired: 3 in, 2 out]
                          n188 = Bundle By Name(cluster=w872, "State"=w874, "Stack Number"=w873, "Image"=w870) -> (w875:T3)
                          n189 = Enqueue Element(queue=w876, element=w875) -> (queue out=w871:refnum<queue>)  [unwired: 2 in, 2 out]
                        }
                        n190 = call <userlib>:"tm_stopcapture.vi"("error in (no error)"=w859, "Handle in"=w860) -> ("error out"=w857:errorcluster, "Handle out"=w858:u32)  [unwired: 8 in]
                        n191 = call <userlib>:"tm_unpreparecapture.vi"("error in (no error)"=w857, "Handle in"=w858) -> ("error out"=w856:errorcluster, "Handle out"=w855:u32)  [unwired: 8 in]
                        n192 = Enqueue Element(queue=w853, element=T3 {"State"=enum."End", "Stack Number"=0, "Image"=[], "Stacks"=0} ("input cluster")) -> (queue out=w847:refnum<queue>)  [unwired: 2 in, 2 out]
                        n193 = call <userlib>:"tm_preparecapture.vi"("error in (no error)"=w856, "Capture mode"=w854, "Handle in"=w855) -> ("error out"=w851:errorcluster, "Buffer Info"=w846:T7, "Handle out"=w850:u32)  [unwired: 5 in, 1 out]
                        n194 = call <userlib>:"tm_startcapture_b.vi"("error in (no error)"=w851, "Handle in"=w850) -> ("error out"=w848:errorcluster, "Handle out"=w849:u32)  [unwired: 8 in]
                      }
                      frame Error {
                        w894 = 1 items=["Snap", "Sequence"] ("Capture mode")
                        # "Prepare camera failure, likely too many frames in stack"
                        n195 = One Button Dialog(message="Too many frames in stack", button name ("OK")="OK") -> (true=w899:bool)
                        n196 = call <userlib>:"tm_stopcapture.vi"("error in (no error)"=w890, "Handle in"=w891) -> ("error out"=w897:errorcluster, "Handle out"=w898:u32)  [unwired: 8 in]
                        n197 = call <userlib>:"tm_unpreparecapture.vi"("error in (no error)"=w897, "Handle in"=w898) -> ("error out"=w896:errorcluster, "Handle out"=w895:u32)  [unwired: 8 in]
                        n198 = Enqueue Element(queue=w885, element=T3 {"State"=enum."Idle", "Stack Number"=0, "Image"=[], "Stacks"=0} ("input cluster")) -> ()  [unwired: 2 in, 3 out]
                        n199 = call <userlib>:"tm_preparecapture.vi"("error in (no error)"=w896, "Capture mode"=w894, "Handle in"=w895) -> ("error out"=w893:errorcluster, "Buffer Info"=w888:T7, "Handle out"=w892:u32)  [unwired: 5 in, 1 out]
                        n200 = call <userlib>:"tm_startcapture_b.vi"("error in (no error)"=w893, "Handle in"=w892) -> ("error out"=w889:errorcluster, "Handle out"=w887:u32)  [unwired: 8 in]
                      }
                    }
                  }
                }
              }
              event "HardDisk Record": Value Change {
                n201 = event-data() -> ()  [unwired: 1 in, 5 out]
                n202 = case shown="True" "HardDisk Record" {
                  tunnel: w914 -> [w917 w933]
                  tunnel: w913 -> [w916 w930]
                  tunnel: [w917 w920] -> w912
                  tunnel: [w916 w922] -> w911
                  tunnel: [w915 w921] -> w907
                  tunnel: w906 -> [w915 _]
                  tunnel: w904 -> [_ w918]
                  tunnel: [_ w923] -> w903
                  frame False {
                  }
                  frame True {
                    w927 = 0 items=["Snap", "Sequence"] ("Capture mode")
                    # "Max 50"
                    n203 = call <userlib>:"tm_stopcapture.vi"("error in (no error)"=w933, "Handle in"=w930) -> ("error out"=w932:errorcluster, "Handle out"=w931:u32)  [unwired: 8 in]
                    n204 = call <userlib>:"tm_unpreparecapture.vi"("error in (no error)"=w932, "Handle in"=w931) -> ("error out"=w928:errorcluster, "Handle out"=w929:u32)  [unwired: 8 in]
                    n205 = call <userlib>:"tm_preparecapture.vi"("error in (no error)"=w928, "Frames"="Frames", "Capture mode"=w927, "Handle in"=w929) -> ("error out"=w926:errorcluster, "Buffer Info"=w924:T7, "Handle out"=w925:u32)  [unwired: 4 in, 1 out]
                    n206 = case shown="No Error" w926 {
                      selector: w926 -> [w958 w971]
                      tunnel: w925 -> [w944 w972]
                      tunnel: [w947 w968] -> w922
                      tunnel: w924 -> [w955 _]
                      tunnel: [w946 w970] -> w920
                      tunnel: [FALSE ("value") w980] -> w923
                      tunnel: [w945 w969] -> w921
                      tunnel: "Frames" -> [w941 _]
                      tunnel: w918 -> [w935 w966]
                      frame No Error {
                        w950 = 1 items=["Snap", "Sequence"] ("Capture mode")
                        n207 = call <userlib>:"tm_startrecorder.vi"("frames"=w941, "File"="Temp", "Handle in"=w944) -> ("Handle out"=w943:u32)  [unwired: 7 in, 1 out]
                        n208 = call <userlib>:"tm_startcapture_b.vi"("error in (no error)"=w958, "Handle in"=w943) -> ("error out"=w956:errorcluster, "Handle out"=w957:u32)  [unwired: 8 in]
                        n209 = while {
                          tunnel: w957 -> [w964]
                          tunnel: w956 -> [w963]
                          tunnel: w955 -> [_]
                          tunnel: [w965] -> w953
                          tunnel: w941 -> [w960]
                          stop <- w961 stop-if-true
                          n210 = Wait (ms)(milliseconds to wait=u32 50) -> ()  [unwired: 1 out]
                          n211 = call <userlib>:"tm_getrecorderstatus.vi"("error in (no error)"=w963, "Handle"=w964) -> ("error out"=w965:errorcluster, "Count"=w959:i32)  [unwired: 6 in, 2 out]
                          n212 = Equal?(x=w959, y=w960) -> (x = y?=w961:bool)
                        }
                        n213 = call <userlib>:"tm_stopcapture.vi"("error in (no error)"=w953) -> ("error out"=w940:errorcluster, "Handle out"=w939:u32)  [unwired: 9 in]
                        n214 = call <userlib>:"tm_stoprecorder.vi"("error in (no error)"=w940, "Handle in"=w939) -> ("error out"=w937:errorcluster, "Handle out"=w938:u32)  [unwired: 8 in]
                        n215 = Enqueue Element(queue=w935, element=T3 {"State"=enum."Read Disk", "Stack Number"=0, "Image"=[], "Stacks"=0}, error in (no error)=w937) -> (error out=w936:errorcluster)  [unwired: 1 in, 2 out]
                        n216 = call <userlib>:"tm_unpreparecapture.vi"("error in (no error)"=w936, "Handle in"=w938) -> ("error out"=w952:errorcluster, "Handle out"=w951:u32)  [unwired: 8 in]
                        n217 = call <userlib>:"tm_preparecapture.vi"("error in (no error)"=w952, "Capture mode"=w950, "Handle in"=w951) -> ("error out"=w949:errorcluster, "Buffer Info"=w945:T7, "Handle out"=w948:u32)  [unwired: 5 in, 1 out]
                        n218 = call <userlib>:"tm_startcapture_b.vi"("error in (no error)"=w949, "Handle in"=w948) -> ("error out"=w946:errorcluster, "Handle out"=w947:u32)  [unwired: 8 in]
                      }
                      frame Error {
                        w975 = 1 items=["Snap", "Sequence"] ("Capture mode")
                        # "Prepare camera failure, likely too many frames in stack"
                        n219 = One Button Dialog(message="Too many frames in stack", button name ("OK")="OK") -> (true=w980:bool)
                        n220 = call <userlib>:"tm_stopcapture.vi"("error in (no error)"=w971, "Handle in"=w972) -> ("error out"=w978:errorcluster, "Handle out"=w979:u32)  [unwired: 8 in]
                        n221 = call <userlib>:"tm_unpreparecapture.vi"("error in (no error)"=w978, "Handle in"=w979) -> ("error out"=w977:errorcluster, "Handle out"=w976:u32)  [unwired: 8 in]
                        n222 = Enqueue Element(queue=w966, element=T3 {"State"=enum."STOP", "Stack Number"=0, "Image"=[], "Stacks"=0} ("input cluster")) -> ()  [unwired: 2 in, 3 out]
                        n223 = call <userlib>:"tm_preparecapture.vi"("error in (no error)"=w977, "Capture mode"=w975, "Handle in"=w976) -> ("error out"=w974:errorcluster, "Buffer Info"=w969:T7, "Handle out"=w973:u32)  [unwired: 5 in, 1 out]
                        n224 = call <userlib>:"tm_startcapture_b.vi"("error in (no error)"=w974, "Handle in"=w973) -> ("error out"=w970:errorcluster, "Handle out"=w968:u32)  [unwired: 8 in]
                      }
                    }
                  }
                }
              }
              event "Scan Mode": Value Change {
                w983 = u32 4211872 items=["SENSOR MODE"=4212128, "CCD MODE"=4212384, "READOUT MODE"=4211872, "ACTIVE VIEW INDEX"=4343136, "BITS PER CHANNEL"=4342976, "IMAGE PIXEL TYPE"=4343296, "BINNING"=4215968, "EXPOSURE TIME"=2049184, "CONTRAST GAIN"=3163312, "CONTRAST OFFSET"=3163328, "LIGHT MODE"=2114720, "SENSITIVITY"=2114992, "PHOTON IMAGING MODE"=2115200, "HIGH DYNAMIC RANGE MODE"=3163360, "WHITE BALANCE"=3163568, "TEMPERATURE"=2115232, "TEMPERATURE TARGET"=2115264, "SENSOR COOLER FAN"=2115296, "LINEBUNDLE HEIGHT"=4212192, "MECHANICAL SHUTTER"=2115488, "BACK FOCUS POSITION"=8422304, "TRIGGER CONNECTOR"=1066432, "TRIGGER SOURCE"=1066144, "OUTPUT TRIGGER SOURCE"=1852576, "TRIGGER GLOBAL EXPOSURE"=2049680, "FIRST TRIGGER BEHAVIOR"=2049696, "CHANNEL SYNC"=1852352, "READOUT DIRECTION"=4211904, "PRE HSYNC COUNT"=1852704] ("Parameter")
                w998 = 1 items=["Snap", "Sequence"] ("Capture mode")
                n225 = event-data() -> ("NewVal"=w988:dbl)  [unwired: 1 in, 2 out]
                n226 = call <userlib>:"tm_stopcapture.vi"("error in (no error)"=w999, "Handle in"=w1000) -> ("error out"=w1001:errorcluster, "Handle out"=w1002:u32)  [unwired: 8 in]
                n227 = call <userlib>:"tm_unpreparecapture.vi"("error in (no error)"=w1001, "Handle in"=w1002) -> ("error out"=w986:errorcluster, "Handle out"=w987:u32)  [unwired: 8 in]
                n228 = call <userlib>:"tm_setparameter_a.vi"("error in (no error)"=w986, "Value in"=w988, "Parameter"=w983, "Handle in"=w987) -> ("error out"=w985:errorcluster, "Handle out"=w984:u32)  [unwired: 6 in]
                n229 = call <userlib>:"tm_getparameter_a.vi"("error in (no error)"=w985, "Parameter"=w983, "Handle in"=w984) -> ("error out"=w991:errorcluster, "Value out"=w990:dbl, "Handle out"=w989:u32)  [unwired: 6 in]
                n230 = local write "SMD"(w990) -> ()
                n231 = call <userlib>:"tm_preparecapture.vi"("error in (no error)"=w991, "Capture mode"=w998, "Handle in"=w989) -> ("error out"=w996:errorcluster, "Buffer Info"=w993:T7, "Handle out"=w997:u32)  [unwired: 5 in, 1 out]
                n232 = call <userlib>:"tm_startcapture_b.vi"("error in (no error)"=w996, "Handle in"=w997) -> ("error out"=w995:errorcluster, "Handle out"=w994:u32)  [unwired: 8 in]
              }
              event "Binning": Value Change {
                w1007 = u32 4215968 items=["BINNING"=4215968, "BITS PER CHANNEL"=2, "ACTIVE VIEW INDEX"=3, "CCD MODE"=4, "SENSOR MODE"=5, "READOUT MODE"=6, "EXPOSURE TIME"=7, "CONTRAST GAIN"=8, "CONTRAST OFFSET"=9, "LIGHT MODE"=10, "SENSITIVITY"=11, "WHITE BALANCE"=12, "PHOTON IMAGING MODE"=13, "HIGH DYNAMIC RANGE MODE"=14, "TRIGGER SOURCE"=15, "TRIGGER ACTIVE"=16, "TRIGGER MODE"=17, "TRIGGER POLARITY"=18, "TRIGGER GLOBAL EXPOSURE"=19, "FIRST TRIGGER BEHAVIOR"=20, "TRIGGER TIMES"=21, "OUTPUT TRIGGER POLARITY"=22, "OUTPUT TRIGGER DELAY"=23, "OUTPUT TRIGGER PERIOD"=24, "TEMPERATURE"=25, "TEMPERATURE TARGET"=26, "SENSOR COOLER FAN"=27, "MECHANICAL SHUTTER"=28, "BACK FOCUS POSITION"=29, "FRAMEBUNDLE MODE"=30, "FRAMEBUNDLE NUMBER"=31, "LINEBUNDLE HEIGHT"=32, "TRIGGER CONNECTOR"=33, "IMAGE PIXEL TYPE"=34, "OUTPUT TRIGGER KIND"=35, "READOUT DIRECTION"=36, "CHANNEL SYNC"=37] ("Parameter")
                w1046 = 1 items=["Snap", "Sequence"] ("Capture mode")
                n233 = event-data() -> ("NewVal"=w1008:u16)  [unwired: 1 in, 2 out]
                n234 = call <userlib>:"tm_stopcapture.vi"("error in (no error)"=w1015, "Handle in"=w1016) -> ("error out"=w1013:errorcluster, "Handle out"=w1014:u32)  [unwired: 8 in]
                n235 = call <userlib>:"tm_unpreparecapture.vi"("error in (no error)"=w1013, "Handle in"=w1014) -> ("error out"=w1009:errorcluster, "Handle out"=w1006:u32)  [unwired: 8 in]
                n236 = call <userlib>:"tm_setparameter_a.vi"("error in (no error)"=w1009, "Value in"=w1008, "Parameter"=w1007, "Handle in"=w1006) -> ("error out"=w1010:errorcluster, "Handle out"=w1011:u32)  [unwired: 6 in]
                n237 = call <userlib>:"tm_getarea_a.vi"("error in (no error)"=w1010, "Handle in"=w1011) -> ("error out"=w1034:errorcluster, "V Offset"=w1036:T6, "H Offset"=w1035:T6, "Handle out"=w1033:u32, "H Width"=w1037:T6, "V Width"=w1038:T6)  [unwired: 4 in]
                n238 = Unbundle By Name(w1035) -> ("Value"=w1029:i32, "Minimum"=w1032:i32, "Maximum"=w1031:i32, "Increment"=w1030:i32)
                n239 = Unbundle By Name(w1036) -> ("Value"=w1019:i32, "Minimum"=w1028:i32, "Maximum"=w1027:i32, "Increment"=w1026:i32)
                n240 = Unbundle By Name(w1037) -> ("Value"=w1018:i32, "Minimum"=w1025:i32, "Maximum"=w1024:i32, "Increment"=w1023:i32)
                n241 = Unbundle By Name(w1038) -> ("Value"=w1017:i32, "Minimum"=w1022:i32, "Maximum"=w1021:i32, "Increment"=w1020:i32)
                n242 = property on="H Offset" class="DigNum (strict)"("Value"=w1029, "Minimum"=w1032, "Maximum"=w1031, "Increment"=w1030) -> ()  [unwired: 2 in, 2 out]
                n243 = property on="V Offset" class="DigNum (strict)"("Value"=w1019, "Minimum"=w1028, "Maximum"=w1027, "Increment"=w1026) -> ()  [unwired: 2 in, 2 out]
                n244 = property on="H Width" class="DigNum (strict)"("Value"=w1018, "Minimum"=w1025, "Maximum"=w1024, "Increment"=w1023) -> ()  [unwired: 2 in, 2 out]
                n245 = property on="V Width" class="DigNum (strict)"("Value"=w1017, "Minimum"=w1022, "Maximum"=w1021, "Increment"=w1020) -> ()  [unwired: 2 in, 2 out]
                n246 = local write "SHO"(w1029) -> ()
                n247 = local write "SVO"(w1019) -> ()
                n248 = local write "SHW"(w1018) -> ()
                n249 = local write "SVW"(w1017) -> ()
                n250 = call <userlib>:"tm_preparecapture.vi"("error in (no error)"=w1034, "Capture mode"=w1046, "Handle in"=w1033) -> ("error out"=w1044:errorcluster, "Buffer Info"=w1041:T7, "Handle out"=w1045:u32)  [unwired: 5 in, 1 out]
                n251 = call <userlib>:"tm_startcapture_b.vi"("error in (no error)"=w1044, "Handle in"=w1045) -> ("error out"=w1043:errorcluster, "Handle out"=w1042:u32)  [unwired: 8 in]
              }
              event "H Offset", "H Width", "V Offset", "V Width": Value Change {
                w1091 = 1 items=["Snap", "Sequence"] ("Capture mode")
                n252 = event-data() -> ()  [unwired: 1 in, 4 out]
                n253 = call <userlib>:"tm_stopcapture.vi"("error in (no error)"=w1053, "Handle in"=w1054) -> ("error out"=w1051:errorcluster, "Handle out"=w1052:u32)  [unwired: 8 in]
                n254 = local read "H Offset"() -> (w1057:i32)
                n255 = local read "H Width"() -> (w1058:i32)
                n256 = local read "V Offset"() -> (w1059:i32)
                n257 = local read "V Width"() -> (w1056:i32)
                n258 = call <userlib>:"tm_unpreparecapture.vi"("error in (no error)"=w1051, "Handle in"=w1052) -> ("error out"=w1049:errorcluster, "Handle out"=w1050:u32)  [unwired: 8 in]
                n259 = Bundle("H Offset"=w1057, "V Offset"=w1059, "H Width"=w1058, "V Width"=w1056) -> (w1055:T8)  [unwired: 1 in]
                n260 = call <userlib>:"tm_setarea.vi"("error in (no error)"=w1049, "Sub Region"=w1055, "Handle in"=w1050) -> ("error out"=w1060:errorcluster, "Handle out"=w1061:u32)  [unwired: 7 in]
                n261 = call <userlib>:"tm_getarea_a.vi"("error in (no error)"=w1060, "Handle in"=w1061) -> ("error out"=w1079:errorcluster, "V Offset"=w1081:T6, "H Offset"=w1080:T6, "Handle out"=w1078:u32, "H Width"=w1082:T6, "V Width"=w1083:T6)  [unwired: 4 in]
                n262 = Unbundle By Name(w1080) -> ("Value"=w1074:i32, "Minimum"=w1077:i32, "Maximum"=w1076:i32, "Increment"=w1075:i32)
                n263 = Unbundle By Name(w1081) -> ("Value"=w1064:i32, "Minimum"=w1073:i32, "Maximum"=w1072:i32, "Increment"=w1071:i32)
                n264 = Unbundle By Name(w1082) -> ("Value"=w1063:i32, "Minimum"=w1070:i32, "Maximum"=w1069:i32, "Increment"=w1068:i32)
                n265 = Unbundle By Name(w1083) -> ("Value"=w1062:i32, "Minimum"=w1067:i32, "Maximum"=w1066:i32, "Increment"=w1065:i32)
                n266 = property on="H Offset" class="DigNum (strict)"("Value"=w1074, "Minimum"=w1077, "Maximum"=w1076, "Increment"=w1075) -> ()  [unwired: 2 in, 2 out]
                n267 = property on="V Offset" class="DigNum (strict)"("Value"=w1064, "Minimum"=w1073, "Maximum"=w1072, "Increment"=w1071) -> ()  [unwired: 2 in, 2 out]
                n268 = property on="H Width" class="DigNum (strict)"("Value"=w1063, "Minimum"=w1070, "Maximum"=w1069, "Increment"=w1068) -> ()  [unwired: 2 in, 2 out]
                n269 = property on="V Width" class="DigNum (strict)"("Value"=w1062, "Minimum"=w1067, "Maximum"=w1066, "Increment"=w1065) -> ()  [unwired: 2 in, 2 out]
                n270 = local write "SHO"(w1074) -> ()
                n271 = local write "SVO"(w1064) -> ()
                n272 = local write "SHW"(w1063) -> ()
                n273 = local write "SVW"(w1062) -> ()
                n274 = call <userlib>:"tm_preparecapture.vi"("error in (no error)"=w1079, "Capture mode"=w1091, "Handle in"=w1078) -> ("error out"=w1089:errorcluster, "Buffer Info"=w1086:T7, "Handle out"=w1090:u32)  [unwired: 5 in, 1 out]
                n275 = call <userlib>:"tm_startcapture_b.vi"("error in (no error)"=w1089, "Handle in"=w1090) -> ("error out"=w1088:errorcluster, "Handle out"=w1087:u32)  [unwired: 8 in]
              }
            }
            n276 = local read "stop"() -> (w595:bool)
            n277 = Unbundle By Name(w604) -> ("status"=w617:bool)
            n278 = Compound Arithmetic op=OR(w617, w595, w599) -> (w616:bool)
          }
        }
        frame Enabled {
        }
      }
      n279 = while {
        tunnel: w16 -> [w167]
        tunnel: w19 -> [w170]
        tunnel: w30 -> [w166]
        shift-right: [w165] -> _
        shift-left: w29 -> [w168]
        shift-right: [w164] -> w25
        shift-left: w28 -> [w169]
        tunnel: w27 -> [w163]
        tunnel: [w157] -> w24
        shift-right: [w155] -> _
        shift-left: _ -> [w154]
        shift-right: [w153] -> _
        shift-left: CameraControlTypeDef."Preview" ("Enum") -> [w152]
        stop <- w156 stop-if-true
        n280 = Dequeue Element(queue=w170, timeout in ms (-1)=1) -> (element=w159:T2, timed out?=w161:bool)  [unwired: 1 in, 2 out]
        n281 = case shown="True" w161 {
          tunnel: [w171 w172] -> w160
          tunnel: w159 -> [w171 _]
          tunnel: w152 -> [_ w172]
          frame False {
          }
          frame True {
          }
        }
        n282 = case shown="\"Trigger Mode\"" w160 {
          tunnel: w169 -> [w191 w276 w334 w377 w417 w455 w490 w494 w512 w523 w557 w578 w582]
          tunnel: w168 -> [_ _ _ _ _ w462 w484 w495 _ _ _ _ w581]
          tunnel: w167 -> [w193 w277 _ _ _ _ w489 _ _ _ _ _ _]
          tunnel: w166 -> [w194 w260 _ _ _ _ w488 _ _ _ _ _ _]
          tunnel: [w178 w268 w347 w386 w424 w462 w484 w495 w498 w521 w541 w562 w581] -> w165
          tunnel: [w173 w267 w340 w384 w422 w463 w483 w494 w502 w520 w553 w574 w582] -> w164
          tunnel: w163 -> [w192 w275 w372 w412 w432 w454 w481 w493 w515 w522 w547 w568 w583]
          tunnel: [w179 w264 w346 w385 w423 w461 w482 w493 w503 w519 w552 w573 w583] -> w157
          tunnel: [w184 w270 w333 w376 w416 w453 w480 w492 w497 w518 w539 w560 w580] -> w155
          tunnel: w154 -> [w183 w270 w333 w376 w416 w453 _ w492 w497 w518 w539 w560 w580]
          tunnel: [w182 w269 w332 w375 w415 w452 CameraControlTypeDef."Preview" ("Enum") CameraControlTypeDef."Idle" ("Enum") w496 w517 w538 w559 w579] -> w153
          tunnel: w152 -> [w182 w269 w332 w375 w415 w452 _ _ w496 w517 w538 w559 w579]
          frame "Ram Record" {
            w177 = 1 items=["Snap", "Sequence"] ("Capture mode")
            n283 = call <userlib>:"tm_stopcapture.vi"("error in (no error)"=w192, "Handle in"=w191) -> ("error out"=w190:errorcluster, "Handle out"=w189:u32)  [unwired: 8 in]
            n284 = local read "Stacks"() -> (w176:dbl)
            n285 = call <userlib>:"tm_unpreparecapture.vi"("error in (no error)"=w190, "Handle in"=w189) -> ("error out"=w187:errorcluster, "Handle out"=w188:u32)  [unwired: 8 in]
            n286 = Flush Queue(queue=w193) -> (queue out=w186:refnum<queue>)  [unwired: 1 in, 2 out]
            n287 = for {
              N: w176 -> [_]
              tunnel: w194 -> [w215]
              tunnel: w186 -> [w207]
              tunnel: [w202] -> w185
              tunnel: [w201] -> w184
              tunnel: w183 -> [w200]
              shift-right: [w197] -> w174
              shift-left: w188 -> [w214]
              shift-right: [w195] -> w175
              shift-left: w187 -> [w213]
              w212 = 0 items=["Snap", "Sequence"] ("Capture mode")
              # "Max 2500"
              n288 = local read "Stack Frames"() -> (w203:i32)
              n289 = Bundle By Name(cluster=w215, "State"=Stack_Track."Start Sequence", "Stack Number"=0, "Image"=w200) -> (w204:T3)
              n290 = call <userlib>:"tm_preparecapture.vi"("error in (no error)"=w213, "Frames"=w203, "Capture mode"=w212, "Handle in"=w214) -> ("error out"=w211:errorcluster, "Buffer Info"=w209:T7, "Handle out"=w210:u32)  [unwired: 4 in, 1 out]
              n291 = Enqueue Element(queue=w207, element=w204) -> (queue out=w208:refnum<queue>)  [unwired: 2 in, 2 out]
              n292 = case shown="No Error" w211 {
                selector: w211 -> [w233 w250]
                tunnel: w210 -> [w232 w251]
                tunnel: w203 -> [w228 _]
                tunnel: [w217 w251] -> w198
                tunnel: w209 -> [w229 _]
                tunnel: [w216 w250] -> w196
                tunnel: w208 -> [w227 w253]
                tunnel: w215 -> [w226 _]
                tunnel: [w222 w253] -> _
                tunnel: [FALSE ("value") w255] -> _
                tunnel: [FALSE ("Boolean") _] -> w202
                tunnel: [w219 w252] -> w201
                tunnel: w200 -> [_ w252]
                frame No Error {
                  # "Frames in RAM"
                  n293 = call <userlib>:"tm_startcapture_b.vi"("error in (no error)"=w233, "Handle in"=w232) -> ("error out"=w230:errorcluster, "Handle out"=w231:u32)  [unwired: 8 in]
                  n294 = for {
                    N: w228 -> [_]
                    tunnel: w231 -> [w249]
                    tunnel: w230 -> [w248]
                    tunnel: w229 -> [w245]
                    tunnel: [w244] -> w217
                    tunnel: [w243] -> w216
                    tunnel: w227 -> [w242]
                    tunnel: Stack_Track."Collecting" ("Enum") -> [w240]
                    tunnel: w226 -> [w238]
                    tunnel: [w237] -> w224
                    tunnel: [w235] -> w219
                    tunnel: TRUE ("Boolean") -> [w234]
                    i -> [w239]
                    n295 = local write "Record Ready"(w234) -> ()
                    n296 = call <userlib>:"tm_waitnextframe.vi"("error in (no error)"=w248, "Handle in"=w249) -> ("error out"=w246:errorcluster, "Frame Index"=w236:i32, "Handle out"=w247:u32)  [unwired: 6 in, 1 out]
                    n297 = call <userlib>:"tm_getframe_a.vi"("error in (no error)"=w246, "Frame Index"=w239, "Buffer Info"=w245, "Handle in"=w247) -> ("error out"=w243:errorcluster, "Data 16"=w235:u16[][], "Handle out"=w244:u32)  [unwired: 3 in, 2 out]
                    n298 = Bundle By Name(cluster=w238, "State"=w240, "Stack Number"=w239, "Image"=w235) -> (w241:T3)
                    n299 = Enqueue Element(queue=w242, element=w241) -> (queue out=w237:refnum<queue>)  [unwired: 2 in, 2 out]
                    n300 = local write "Stack Frames"(w236) -> ()
                  }
                  n301 = Enqueue Element(queue=w224, element=T3 {"State"=enum."End", "Stack Number"=0, "Image"=[], "Stacks"=0} ("input cluster")) -> (queue out=w222:refnum<queue>)  [unwired: 2 in, 2 out]
                }
                frame Error {
                  # "Prepare camera failure, likely too many frames in stack"
                  n302 = One Button Dialog(message="Too many frames in stack", button name ("OK")="OK") -> (true=w255:bool)
                  n303 = Enqueue Element(queue=w253, element=T3 {"State"=enum."Idle", "Stack Number"=0, "Image"=[], "Stacks"=0} ("input cluster")) -> ()  [unwired: 2 in, 3 out]
                }
              }
              n304 = call <userlib>:"tm_stopcapture.vi"("error in (no error)"=w196, "Handle in"=w198) -> ("error out"=w199:errorcluster)  [unwired: 8 in, 1 out]
              n305 = call <userlib>:"tm_unpreparecapture.vi"("error in (no error)"=w199) -> ("error out"=w195:errorcluster, "Handle out"=w197:u32)  [unwired: 9 in]
            }
            n306 = local write "Record Ready"(w185) -> ()
            n307 = call <userlib>:"tm_preparecapture.vi"("error in (no error)"=w175, "Capture mode"=w177, "Handle in"=w174) -> ("error out"=w180:errorcluster, "Buffer Info"=w178:T7, "Handle out"=w181:u32)  [unwired: 5 in, 1 out]
            n308 = call <userlib>:"tm_startcapture_b.vi"("error in (no error)"=w180, "Handle in"=w181) -> ("error out"=w179:errorcluster, "Handle out"=w173:u32)  [unwired: 8 in]
          }
          frame "HardDisk Record" {
            w263 = 1 items=["Snap", "Sequence"] ("Capture mode")
            n309 = local read "Stacks"() -> (w262:dbl)
            n310 = call <userlib>:"tm_stopcapture.vi"("error in (no error)"=w275, "Handle in"=w276) -> ("error out"=w274:errorcluster, "Handle out"=w273:u32)  [unwired: 8 in]
            n311 = call <userlib>:"tm_unpreparecapture.vi"("error in (no error)"=w274, "Handle in"=w273) -> ("error out"=w271:errorcluster, "Handle out"=w272:u32)  [unwired: 8 in]
            n312 = for {
              N: w262 -> [_]
              tunnel: w277 -> [w299]
              shift-right: [w281] -> w258
              shift-left: w272 -> [w298]
              shift-right: [w282] -> w259
              shift-left: w271 -> [w297]
              tunnel: path "C:/temp" ("Temp 2") -> [w287]
              tunnel: w260 -> [w289]
              i -> [w285]
              w296 = 0 items=["Snap", "Sequence"] ("Capture mode")
              # "Would add for loop here"
              # "Max 50"
              n313 = local read "Stack Frames"() -> (w293:i32)
              n314 = call "4Digit File Incrementer tmp.vi"("Number"=w285, "path"=w287) -> ("appended path"=w286:path)  [unwired: 9 in]
              n315 = call <userlib>:"tm_preparecapture.vi"("error in (no error)"=w297, "Frames"=w293, "Capture mode"=w296, "Handle in"=w298) -> ("error out"=w295:errorcluster, "Buffer Info"=w294:T7, "Handle out"=w284:u32)  [unwired: 4 in, 1 out]
              n316 = Bundle By Name(cluster=w289, "State"=Stack_Track."Read Disk", "Stack Number"=0, "Image"=u16[][] [], "Stacks"=w285) -> (w288:T3)
              n317 = case shown="No Error" w295 {
                selector: w295 -> [w305 w325]
                tunnel: w284 -> [w312 w326]
                tunnel: w294 -> [w314 _]
                tunnel: [FALSE ("value") w329] -> _
                tunnel: w293 -> [w310 _]
                tunnel: w299 -> [w308 w327]
                tunnel: w286 -> [w306 _]
                tunnel: [w304 w325] -> w278
                tunnel: [w303 w326] -> w279
                tunnel: w288 -> [w300 _]
                frame No Error {
                  n318 = call <userlib>:"tm_startrecorder.vi"("error in (no error)"=w305, "frames"=w310, "File"=w306, "Handle in"=w312) -> ("error out"=w307:errorcluster, "Handle out"=w311:u32)  [unwired: 6 in]
                  n319 = call <userlib>:"tm_startcapture_b.vi"("error in (no error)"=w307, "Handle in"=w311) -> ("error out"=w315:errorcluster, "Handle out"=w316:u32)  [unwired: 8 in]
                  n320 = while {
                    tunnel: w316 -> [w323]
                    tunnel: w315 -> [w322]
                    tunnel: w314 -> [_]
                    tunnel: [w324] -> w301
                    tunnel: w310 -> [w319]
                    tunnel: [w317] -> w302
                    stop <- w320 stop-if-true
                    n321 = Wait (ms)(milliseconds to wait=u32 50) -> ()  [unwired: 1 out]
                    n322 = call <userlib>:"tm_getrecorderstatus.vi"("error in (no error)"=w322, "Handle"=w323) -> ("error out"=w324:errorcluster, "Count"=w318:i32, "Handle"=w317:u32)  [unwired: 6 in, 1 out]
                    n323 = Equal?(x=w318, y=w319) -> (x = y?=w320:bool)
                  }
                  n324 = call <userlib>:"tm_stoprecorder.vi"("error in (no error)"=w301, "Handle in"=w302) -> ("error out"=w309:errorcluster, "Handle out"=w303:u32)  [unwired: 8 in]
                  n325 = Enqueue Element(queue=w308, element=w300, error in (no error)=w309) -> (error out=w304:errorcluster)  [unwired: 1 in, 2 out]
                }
                frame Error {
                  # "Prepare camera failure, likely too many frames in stack"
                  n326 = One Button Dialog(message="Too many frames in stack", button name ("OK")="OK") -> (true=w329:bool)
                  n327 = Enqueue Element(queue=w327, element=T3 {"State"=enum."STOP", "Stack Number"=0, "Image"=[], "Stacks"=0} ("input cluster")) -> ()  [unwired: 2 in, 3 out]
                }
              }
              n328 = call <userlib>:"tm_stopcapture.vi"("error in (no error)"=w278, "Handle in"=w279) -> ("error out"=w283:errorcluster, "Handle out"=w280:u32)  [unwired: 8 in]
              n329 = call <userlib>:"tm_unpreparecapture.vi"("error in (no error)"=w283, "Handle in"=w280) -> ("error out"=w282:errorcluster, "Handle out"=w281:u32)  [unwired: 8 in]
            }
            n330 = call <userlib>:"tm_preparecapture.vi"("error in (no error)"=w259, "Capture mode"=w263, "Handle in"=w258) -> ("error out"=w265:errorcluster, "Buffer Info"=w268:T7, "Handle out"=w266:u32)  [unwired: 5 in, 1 out]
            n331 = call <userlib>:"tm_startcapture_b.vi"("error in (no error)"=w265, "Handle in"=w266) -> ("error out"=w264:errorcluster, "Handle out"=w267:u32)  [unwired: 8 in]
          }
          frame "ROI" {
            w350 = 1 items=["Snap", "Sequence"] ("Capture mode")
            n332 = call <userlib>:"tm_stopcapture.vi"("error in (no error)"=w372, "Handle in"=w334) -> ("error out"=w373:errorcluster, "Handle out"=w374:u32)  [unwired: 8 in]
            n333 = call <userlib>:"tm_unpreparecapture.vi"("error in (no error)"=w373, "Handle in"=w374) -> ("error out"=w336:errorcluster, "Handle out"=w337:u32)  [unwired: 8 in]
            n334 = local read "V Width"() -> (w342:i32)
            n335 = local read "V Offset"() -> (w344:i32)
            n336 = local read "H Width"() -> (w343:i32)
            n337 = local read "H Offset"() -> (w345:i32)
            n338 = Bundle("H Offset"=w345, "V Offset"=w344, "H Width"=w343, "V Width"=w342) -> (w341:T8)  [unwired: 1 in]
            n339 = call <userlib>:"tm_setarea.vi"("error in (no error)"=w336, "Sub Region"=w341, "Handle in"=w337) -> ("error out"=w339:errorcluster, "Handle out"=w338:u32)  [unwired: 7 in]
            n340 = call <userlib>:"tm_getarea_a.vi"("error in (no error)"=w339, "Handle in"=w338) -> ("error out"=w351:errorcluster, "V Offset"=w354:T6, "H Offset"=w355:T6, "Handle out"=w335:u32, "H Width"=w353:T6, "V Width"=w352:T6)  [unwired: 4 in]
            n341 = Unbundle By Name(w355) -> ("Value"=w359:i32, "Minimum"=w356:i32, "Maximum"=w357:i32, "Increment"=w358:i32)
            n342 = Unbundle By Name(w354) -> ("Value"=w369:i32, "Minimum"=w360:i32, "Maximum"=w361:i32, "Increment"=w362:i32)
            n343 = Unbundle By Name(w353) -> ("Value"=w370:i32, "Minimum"=w363:i32, "Maximum"=w364:i32, "Increment"=w365:i32)
            n344 = Unbundle By Name(w352) -> ("Value"=w371:i32, "Minimum"=w366:i32, "Maximum"=w367:i32, "Increment"=w368:i32)
            n345 = property on="H Offset" class="DigNum (strict)"("Value"=w359, "Minimum"=w356, "Maximum"=w357, "Increment"=w358) -> ()  [unwired: 2 in, 2 out]
            n346 = property on="V Offset" class="DigNum (strict)"("Value"=w369, "Minimum"=w360, "Maximum"=w361, "Increment"=w362) -> ()  [unwired: 2 in, 2 out]
            n347 = property on="H Width" class="DigNum (strict)"("Value"=w370, "Minimum"=w363, "Maximum"=w364, "Increment"=w365) -> ()  [unwired: 2 in, 2 out]
            n348 = property on="V Width" class="DigNum (strict)"("Value"=w371, "Minimum"=w366, "Maximum"=w367, "Increment"=w368) -> ()  [unwired: 2 in, 2 out]
            n349 = local write "SHO"(w359) -> ()
            n350 = local write "SVO"(w369) -> ()
            n351 = local write "SHW"(w370) -> ()
            n352 = local write "SVW"(w371) -> ()
            n353 = call <userlib>:"tm_preparecapture.vi"("error in (no error)"=w351, "Capture mode"=w350, "Handle in"=w335) -> ("error out"=w349:errorcluster, "Buffer Info"=w347:T7, "Handle out"=w348:u32)  [unwired: 5 in, 1 out]
            n354 = call <userlib>:"tm_startcapture_b.vi"("error in (no error)"=w349, "Handle in"=w348) -> ("error out"=w346:errorcluster, "Handle out"=w340:u32)  [unwired: 8 in]
          }
          frame "Binning" {
            w389 = 1 items=["Snap", "Sequence"] ("Capture mode")
            w379 = u32 4215968 items=["BINNING"=4215968, "BITS PER CHANNEL"=2, "ACTIVE VIEW INDEX"=3, "CCD MODE"=4, "SENSOR MODE"=5, "READOUT MODE"=6, "EXPOSURE TIME"=7, "CONTRAST GAIN"=8, "CONTRAST OFFSET"=9, "LIGHT MODE"=10, "SENSITIVITY"=11, "WHITE BALANCE"=12, "PHOTON IMAGING MODE"=13, "HIGH DYNAMIC RANGE MODE"=14, "TRIGGER SOURCE"=15, "TRIGGER ACTIVE"=16, "TRIGGER MODE"=17, "TRIGGER POLARITY"=18, "TRIGGER GLOBAL EXPOSURE"=19, "FIRST TRIGGER BEHAVIOR"=20, "TRIGGER TIMES"=21, "OUTPUT TRIGGER POLARITY"=22, "OUTPUT TRIGGER DELAY"=23, "OUTPUT TRIGGER PERIOD"=24, "TEMPERATURE"=25, "TEMPERATURE TARGET"=26, "SENSOR COOLER FAN"=27, "MECHANICAL SHUTTER"=28, "BACK FOCUS POSITION"=29, "FRAMEBUNDLE MODE"=30, "FRAMEBUNDLE NUMBER"=31, "LINEBUNDLE HEIGHT"=32, "TRIGGER CONNECTOR"=33, "IMAGE PIXEL TYPE"=34, "OUTPUT TRIGGER KIND"=35, "READOUT DIRECTION"=36, "CHANNEL SYNC"=37] ("Parameter")
            n355 = local read "Binning"() -> (w411:u16)
            n356 = call <userlib>:"tm_stopcapture.vi"("error in (no error)"=w412, "Handle in"=w377) -> ("error out"=w413:errorcluster, "Handle out"=w414:u32)  [unwired: 8 in]
            n357 = call <userlib>:"tm_unpreparecapture.vi"("error in (no error)"=w413, "Handle in"=w414) -> ("error out"=w382:errorcluster, "Handle out"=w383:u32)  [unwired: 8 in]
            n358 = call <userlib>:"tm_setparameter_a.vi"("error in (no error)"=w382, "Value in"=w411, "Parameter"=w379, "Handle in"=w383) -> ("error out"=w380:errorcluster, "Handle out"=w378:u32)  [unwired: 6 in]
            n359 = call <userlib>:"tm_getarea_a.vi"("error in (no error)"=w380, "Handle in"=w378) -> ("error out"=w390:errorcluster, "V Offset"=w393:T6, "H Offset"=w394:T6, "Handle out"=w381:u32, "H Width"=w392:T6, "V Width"=w391:T6)  [unwired: 4 in]
            n360 = Unbundle By Name(w394) -> ("Value"=w398:i32, "Minimum"=w395:i32, "Maximum"=w396:i32, "Increment"=w397:i32)
            n361 = Unbundle By Name(w393) -> ("Value"=w408:i32, "Minimum"=w399:i32, "Maximum"=w400:i32, "Increment"=w401:i32)
            n362 = Unbundle By Name(w392) -> ("Value"=w409:i32, "Minimum"=w402:i32, "Maximum"=w403:i32, "Increment"=w404:i32)
            n363 = Unbundle By Name(w391) -> ("Value"=w410:i32, "Minimum"=w405:i32, "Maximum"=w406:i32, "Increment"=w407:i32)
            n364 = property on="H Offset" class="DigNum (strict)"("Value"=w398, "Minimum"=w395, "Maximum"=w396, "Increment"=w397) -> ()  [unwired: 2 in, 2 out]
            n365 = property on="V Offset" class="DigNum (strict)"("Value"=w408, "Minimum"=w399, "Maximum"=w400, "Increment"=w401) -> ()  [unwired: 2 in, 2 out]
            n366 = property on="H Width" class="DigNum (strict)"("Value"=w409, "Minimum"=w402, "Maximum"=w403, "Increment"=w404) -> ()  [unwired: 2 in, 2 out]
            n367 = property on="V Width" class="DigNum (strict)"("Value"=w410, "Minimum"=w405, "Maximum"=w406, "Increment"=w407) -> ()  [unwired: 2 in, 2 out]
            n368 = local write "SHO"(w398) -> ()
            n369 = local write "SVO"(w408) -> ()
            n370 = local write "SHW"(w409) -> ()
            n371 = local write "SVW"(w410) -> ()
            n372 = call <userlib>:"tm_preparecapture.vi"("error in (no error)"=w390, "Capture mode"=w389, "Handle in"=w381) -> ("error out"=w388:errorcluster, "Buffer Info"=w386:T7, "Handle out"=w387:u32)  [unwired: 5 in, 1 out]
            n373 = call <userlib>:"tm_startcapture_b.vi"("error in (no error)"=w388, "Handle in"=w387) -> ("error out"=w385:errorcluster, "Handle out"=w384:u32)  [unwired: 8 in]
          }
          frame "Readout Mode" {
            w427 = 1 items=["Snap", "Sequence"] ("Capture mode")
            n374 = call <userlib>:"tm_stopcapture.vi"("error in (no error)"=w432, "Handle in"=w417) -> ("error out"=w433:errorcluster, "Handle out"=w434:u32)  [unwired: 8 in]
            n375 = call <userlib>:"tm_unpreparecapture.vi"("error in (no error)"=w433, "Handle in"=w434) -> ("error out"=w418:errorcluster, "Handle out"=w419:u32)  [unwired: 8 in]
            n376 = local read "Camera Readout Mode"() -> (w430:u16)
            n377 = call <userlib>:"tm_setpropertyvalue.vi"("error in (no error)"=w418, "Value in"=w430, "Property ID"=u32 4194832, "Handle in"=w419) -> ("error out"=w428:errorcluster, "Handle out"=w429:u32)  [unwired: 6 in]
            n378 = case shown="12" w430 {
              tunnel: [w438 w443] -> w421
              tunnel: w429 -> [w437 w444]
              tunnel: w428 -> [w436 w443]
              tunnel: [w435 w442] -> w420
              frame 1, Default {
                n379 = local read "Exposure"() -> (w439:dbl)
                n380 = call <userlib>:"tm_setpropertyvalue.vi"("error in (no error)"=w436, "Value in"=w439, "Property ID"=u32 2031888, "Handle in"=w437) -> ("error out"=w438:errorcluster, "Handle out"=w435:u32)  [unwired: 6 in]
              }
              frame 12 {
                n381 = local read "Slit Width / Lines"() -> (w441:sgl)
                n382 = local read "Exposure"() -> (w451:dbl)
                n383 = local read "SVW"() -> (w450:i32)
                n384 = formula code="slitExpos=frameInter*LW/(LinesToReadout\n+10+LW);\nlineInter = slitExpos / LW;"("frameInter"=w451, "LW"=w441, "LinesToReadout"=w450) -> ("slitExpos"=w445:dbl, "lineInter"=w448:dbl)
                n385 = call <userlib>:"tm_setpropertyvalue.vi"("Value in"=w448, "Property ID"=u32 4208720, "Handle in"=w444) -> ("Handle out"=w447:u32)  [unwired: 7 in, 1 out]
                n386 = call <userlib>:"tm_setpropertyvalue.vi"("Value in"=w445, "Property ID"=u32 2031888, "Handle in"=w447) -> ("Handle out"=w442:u32)  [unwired: 7 in, 1 out]
              }
            }
            n387 = call <userlib>:"tm_preparecapture.vi"("error in (no error)"=w421, "Capture mode"=w427, "Handle in"=w420) -> ("error out"=w426:errorcluster, "Buffer Info"=w424:T7, "Handle out"=w425:u32)  [unwired: 5 in, 1 out]
            n388 = call <userlib>:"tm_startcapture_b.vi"("error in (no error)"=w426, "Handle in"=w425) -> ("error out"=w423:errorcluster, "Handle out"=w422:u32)  [unwired: 8 in]
          }
          frame "Update" {
            w459 = u32 1066144 items=["SENSOR MODE"=4212128, "CCD MODE"=4212384, "READOUT MODE"=4211872, "ACTIVE VIEW INDEX"=4343136, "BITS PER CHANNEL"=4342976, "IMAGE PIXEL TYPE"=4343296, "BINNING"=4215968, "EXPOSURE TIME"=2049184, "CONTRAST GAIN"=3163312, "CONTRAST OFFSET"=3163328, "LIGHT MODE"=2114720, "SENSITIVITY"=2114992, "PHOTON IMAGING MODE"=2115200, "HIGH DYNAMIC RANGE MODE"=3163360, "WHITE BALANCE"=3163568, "TEMPERATURE"=2115232, "TEMPERATURE TARGET"=2115264, "SENSOR COOLER FAN"=2115296, "LINEBUNDLE HEIGHT"=4212192, "MECHANICAL SHUTTER"=2115488, "BACK FOCUS POSITION"=8422304, "TRIGGER CONNECTOR"=1066432, "TRIGGER SOURCE"=1066144, "OUTPUT TRIGGER SOURCE"=1852576, "TRIGGER GLOBAL EXPOSURE"=2049680, "FIRST TRIGGER BEHAVIOR"=2049696, "CHANNEL SYNC"=1852352, "READOUT DIRECTION"=4211904, "PRE HSYNC COUNT"=1852704] ("Parameter")
            w464 = u32 2049184 items=["SENSOR MODE"=4212128, "CCD MODE"=4212384, "READOUT MODE"=4211872, "ACTIVE VIEW INDEX"=4343136, "BITS PER CHANNEL"=4342976, "IMAGE PIXEL TYPE"=4343296, "BINNING"=4215968, "EXPOSURE TIME"=2049184, "CONTRAST GAIN"=3163312, "CONTRAST OFFSET"=3163328, "LIGHT MODE"=2114720, "SENSITIVITY"=2114992, "PHOTON IMAGING MODE"=2115200, "HIGH DYNAMIC RANGE MODE"=3163360, "WHITE BALANCE"=3163568, "TEMPERATURE"=2115232, "TEMPERATURE TARGET"=2115264, "SENSOR COOLER FAN"=2115296, "LINEBUNDLE HEIGHT"=4212192, "MECHANICAL SHUTTER"=2115488, "BACK FOCUS POSITION"=8422304, "TRIGGER CONNECTOR"=1066432, "TRIGGER SOURCE"=1066144, "OUTPUT TRIGGER SOURCE"=1852576, "TRIGGER GLOBAL EXPOSURE"=2049680, "FIRST TRIGGER BEHAVIOR"=2049696, "CHANNEL SYNC"=1852352, "READOUT DIRECTION"=4211904, "PRE HSYNC COUNT"=1852704] ("Parameter")
            # "Fails"
            # "Error on get"
            n389 = local read "Exposure"() -> (w466:dbl)
            n390 = disable-structure shown="Disabled" {
              disable-tunnel: w455 -> [w471 _]
              disable-tunnel: w454 -> [w470 _]
              frame Disabled {
                w469 = u32 4226016 items=["SENSOR MODE"=4212128, "CCD MODE"=4212384, "READOUT MODE"=4211872, "ACTIVE VIEW INDEX"=4343136, "BITS PER CHANNEL"=4342976, "IMAGE PIXEL TYPE"=4343296, "BINNING"=4215968, "EXPOSURE TIME"=2049184, "CONTRAST GAIN"=3163312, "CONTRAST OFFSET"=3163328, "LIGHT MODE"=2114720, "SENSITIVITY"=2114992, "PHOTON IMAGING MODE"=2115200, "HIGH DYNAMIC RANGE MODE"=3163360, "WHITE BALANCE"=3163568, "TEMPERATURE"=2115232, "TEMPERATURE TARGET"=2115264, "SENSOR COOLER FAN"=2115296, "LINEBUNDLE HEIGHT"=4212192, "MECHANICAL SHUTTER"=2115488, "BACK FOCUS POSITION"=8422304, "TRIGGER CONNECTOR"=1066432, "TRIGGER SOURCE"=1066144, "OUTPUT TRIGGER SOURCE"=1852576, "TRIGGER GLOBAL EXPOSURE"=2049680, "FIRST TRIGGER BEHAVIOR"=2049696, "CHANNEL SYNC"=1852352, "READOUT DIRECTION"=4211904, "PRE HSYNC COUNT"=1852704, "INTERNAL LINE SPEED"=4226000, "INTERNAL LINE INTERVAL"=4226016] ("Parameter")
                n391 = local read "Internal Line Interval"() -> (w473:dbl)
                n392 = call <userlib>:"tm_setparameter_a.vi"("error in (no error)"=w470, "Value in"=w473, "Parameter"=w469, "Handle in"=w471) -> ("error out"=w472:errorcluster, "Handle out"=w475:u32)  [unwired: 6 in]
                n393 = call <userlib>:"tm_getparameter_a.vi"("error in (no error)"=w472, "Parameter"=w469, "Handle in"=w475) -> ("Value out"=w474:dbl)  [unwired: 6 in, 2 out]
                n394 = local write "Internal Line Interval"(w474) -> ()
              }
              frame Enabled {
              }
            }
            n395 = call <userlib>:"tm_setparameter_a.vi"("error in (no error)"=w454, "Value in"=w466, "Parameter"=w464, "Handle in"=w455) -> ("error out"=w468:errorcluster, "Handle out"=w465:u32)  [unwired: 6 in]
            n396 = call <userlib>:"tm_getparameter_a.vi"("error in (no error)"=w468, "Parameter"=w464, "Handle in"=w465) -> ("Value out"=w467:dbl)  [unwired: 6 in, 2 out]
            n397 = local write "EXP"(w467) -> ()
            n398 = local read "Trigger Source"() -> (w457:sgl)
            n399 = call <userlib>:"tm_setparameter_a.vi"("error in (no error)"=w454, "Value in"=w457, "Parameter"=w459, "Handle in"=w455) -> ("error out"=w456:errorcluster, "Handle out"=w460:u32)  [unwired: 6 in]
            n400 = call <userlib>:"tm_getparameter_a.vi"("error in (no error)"=w456, "Parameter"=w459, "Handle in"=w460) -> ("error out"=w461:errorcluster, "Value out"=w458:dbl, "Handle out"=w463:u32)  [unwired: 6 in]
            n401 = local write "Trigger Source"(w458) -> ()
          }
          frame "Preview", Default {
            # "Slows it all down somewhat"
            # "Currently the external trigger setting means that frames are dropped because the system lingers at this point. \nIdeally I should set it so when the system is external and recording it won't run this section.\n\nThis is what HC Image does, it offers no live video when you switch from live to record mode.\n\nRealistically when tirgger set external and this times out once then ignore this step.\nBut it'd have to be reset after a recording.\n\nNeed to think more betterer about how to handle this else frames will just be dropped. Probably best to just have a seperate scan mode\nOr at least just a boolean to turn off this live capture section. Working now maybe"
            n402 = call <userlib>:"tm_waitnextframe.vi"("error in (no error)"=w481, "Timeout"=3000, "Handle in"=w490) -> ("error out"=w477:errorcluster, "Handle out"=w478:u32)  [unwired: 5 in, 2 out]
            n403 = call <userlib>:"tm_getframe_a.vi"("error in (no error)"=w477, "Buffer Info"=w484, "Handle in"=w478) -> ("error out"=w482:errorcluster, "Data 16"=w480:u16[][], "Handle out"=w483:u32)  [unwired: 4 in, 2 out]
            n404 = Bundle By Name(cluster=w488, "State"=Stack_Track."Idle", "Stack Number"=0, "Image"=w480) -> (w485:T3)
            n405 = Enqueue Element(queue=w489, element=w485) -> ()  [unwired: 2 in, 3 out]
          }
          frame "Idle" {
          }
          frame "Scan Mode" {
            w499 = 1 items=["Snap", "Sequence"] ("Capture mode")
            w508 = u32 4211872 items=["SENSOR MODE"=4212128, "CCD MODE"=4212384, "READOUT MODE"=4211872, "ACTIVE VIEW INDEX"=4343136, "BITS PER CHANNEL"=4342976, "IMAGE PIXEL TYPE"=4343296, "BINNING"=4215968, "EXPOSURE TIME"=2049184, "CONTRAST GAIN"=3163312, "CONTRAST OFFSET"=3163328, "LIGHT MODE"=2114720, "SENSITIVITY"=2114992, "PHOTON IMAGING MODE"=2115200, "HIGH DYNAMIC RANGE MODE"=3163360, "WHITE BALANCE"=3163568, "TEMPERATURE"=2115232, "TEMPERATURE TARGET"=2115264, "SENSOR COOLER FAN"=2115296, "LINEBUNDLE HEIGHT"=4212192, "MECHANICAL SHUTTER"=2115488, "BACK FOCUS POSITION"=8422304, "TRIGGER CONNECTOR"=1066432, "TRIGGER SOURCE"=1066144, "OUTPUT TRIGGER SOURCE"=1852576, "TRIGGER GLOBAL EXPOSURE"=2049680, "FIRST TRIGGER BEHAVIOR"=2049696, "CHANNEL SYNC"=1852352, "READOUT DIRECTION"=4211904, "PRE HSYNC COUNT"=1852704] ("Parameter")
            n406 = call <userlib>:"tm_stopcapture.vi"("error in (no error)"=w515, "Handle in"=w512) -> ("error out"=w514:errorcluster, "Handle out"=w513:u32)  [unwired: 8 in]
            n407 = call <userlib>:"tm_unpreparecapture.vi"("error in (no error)"=w514, "Handle in"=w513) -> ("error out"=w510:errorcluster, "Handle out"=w511:u32)  [unwired: 8 in]
            n408 = local read "Scan Mode"() -> (w509:dbl)
            n409 = call <userlib>:"tm_setparameter_a.vi"("error in (no error)"=w510, "Value in"=w509, "Parameter"=w508, "Handle in"=w511) -> ("error out"=w504:errorcluster)  [unwired: 6 in, 1 out]
            n410 = call <userlib>:"tm_getparameter_a.vi"("error in (no error)"=w504, "Parameter"=w508) -> ("error out"=w505:errorcluster, "Value out"=w507:dbl, "Handle out"=w500:u32)  [unwired: 7 in]
            n411 = local write "SMD"(w507) -> ()
            n412 = call <userlib>:"tm_preparecapture.vi"("error in (no error)"=w505, "Capture mode"=w499, "Handle in"=w500) -> ("error out"=w506:errorcluster, "Buffer Info"=w498:T7, "Handle out"=w501:u32)  [unwired: 5 in, 1 out]
            n413 = call <userlib>:"tm_startcapture_b.vi"("error in (no error)"=w506, "Handle in"=w501) -> ("error out"=w503:errorcluster, "Handle out"=w502:u32)  [unwired: 8 in]
          }
          frame "Trigger Mode" {
            w516 = 1 items=["Snap", "Sequence"] ("Capture mode")
            w524 = u32 1049104 ("Property ID")
            n414 = local read "Trigger Mode"() -> (w529:sgl)
            n415 = call <userlib>:"tm_stopcapture.vi"("error in (no error)"=w522, "Handle in"=w523) -> ("error out"=w528:errorcluster, "Handle out"=w536:u32)  [unwired: 8 in]
            n416 = call <userlib>:"tm_unpreparecapture.vi"("error in (no error)"=w528, "Handle in"=w536) -> ("error out"=w526:errorcluster, "Handle out"=w532:u32)  [unwired: 8 in]
            n417 = call <userlib>:"tm_setpropertyvalue.vi"("error in (no error)"=w526, "Value in"=w529, "Property ID"=w524, "Handle in"=w532) -> ("error out"=w525:errorcluster, "Handle out"=w531:u32)  [unwired: 6 in]
            n418 = call <userlib>:"tm_getpropertyvalue.vi"("error in (no error)"=w525, "Property ID"=w524, "Handle in"=w531) -> ("error out"=w533:errorcluster, "Value in"=w530:sgl, "Handle out"=w534:u32)  [unwired: 6 in]
            n419 = local write "Trigger Mode"(w530) -> ()
            n420 = call <userlib>:"tm_preparecapture.vi"("error in (no error)"=w533, "Capture mode"=w516, "Handle in"=w534) -> ("error out"=w527:errorcluster, "Buffer Info"=w521:T7, "Handle out"=w535:u32)  [unwired: 5 in, 1 out]
            n421 = call <userlib>:"tm_startcapture_b.vi"("error in (no error)"=w527, "Handle in"=w535) -> ("error out"=w519:errorcluster, "Handle out"=w520:u32)  [unwired: 8 in]
          }
          frame "Readout Direction" {
            w537 = u32 4211904 items=["SENSOR MODE"=4212128, "CCD MODE"=4212384, "READOUT MODE"=4211872, "ACTIVE VIEW INDEX"=4343136, "BITS PER CHANNEL"=4342976, "IMAGE PIXEL TYPE"=4343296, "BINNING"=4215968, "EXPOSURE TIME"=2049184, "CONTRAST GAIN"=3163312, "CONTRAST OFFSET"=3163328, "LIGHT MODE"=2114720, "SENSITIVITY"=2114992, "PHOTON IMAGING MODE"=2115200, "HIGH DYNAMIC RANGE MODE"=3163360, "WHITE BALANCE"=3163568, "TEMPERATURE"=2115232, "TEMPERATURE TARGET"=2115264, "SENSOR COOLER FAN"=2115296, "LINEBUNDLE HEIGHT"=4212192, "MECHANICAL SHUTTER"=2115488, "BACK FOCUS POSITION"=8422304, "TRIGGER CONNECTOR"=1066432, "TRIGGER SOURCE"=1066144, "OUTPUT TRIGGER SOURCE"=1852576, "TRIGGER GLOBAL EXPOSURE"=2049680, "FIRST TRIGGER BEHAVIOR"=2049696, "CHANNEL SYNC"=1852352, "READOUT DIRECTION"=4211904, "PRE HSYNC COUNT"=1852704, "INTERNAL LINE SPEED"=4226000, "INTERNAL LINE INTERVAL"=4226016] ("Parameter")
            w548 = 1 items=["Snap", "Sequence"] ("Capture mode")
            n422 = call <userlib>:"tm_stopcapture.vi"("error in (no error)"=w547, "Handle in"=w557) -> ("error out"=w549:errorcluster, "Handle out"=w556:u32)  [unwired: 8 in]
            n423 = call <userlib>:"tm_unpreparecapture.vi"("error in (no error)"=w549, "Handle in"=w556) -> ("error out"=w550:errorcluster, "Handle out"=w555:u32)  [unwired: 8 in]
            n424 = local read "Readout Direction"() -> (w540:sgl)
            n425 = call <userlib>:"tm_setparameter_a.vi"("error in (no error)"=w550, "Value in"=w540, "Parameter"=w537, "Handle in"=w555) -> ("error out"=w544:errorcluster, "Handle out"=w546:u32)  [unwired: 6 in]
            n426 = call <userlib>:"tm_getparameter_a.vi"("error in (no error)"=w544, "Parameter"=w537, "Handle in"=w546) -> ("error out"=w543:errorcluster, "Value out"=w542:dbl, "Handle out"=w545:u32)  [unwired: 6 in]
            n427 = local write "Readout Direction"(w542) -> ()
            n428 = call <userlib>:"tm_preparecapture.vi"("error in (no error)"=w543, "Capture mode"=w548, "Handle in"=w545) -> ("error out"=w551:errorcluster, "Buffer Info"=w541:T7, "Handle out"=w554:u32)  [unwired: 5 in, 1 out]
            n429 = call <userlib>:"tm_startcapture_b.vi"("error in (no error)"=w551, "Handle in"=w554) -> ("error out"=w552:errorcluster, "Handle out"=w553:u32)  [unwired: 8 in]
          }
          frame "IntervalLineInt" {
            w558 = 4226016
            w569 = 1 items=["Snap", "Sequence"] ("Capture mode")
            n430 = call <userlib>:"tm_stopcapture.vi"("error in (no error)"=w568, "Handle in"=w578) -> ("error out"=w570:errorcluster, "Handle out"=w577:u32)  [unwired: 8 in]
            n431 = call <userlib>:"tm_unpreparecapture.vi"("error in (no error)"=w570, "Handle in"=w577) -> ("error out"=w571:errorcluster, "Handle out"=w576:u32)  [unwired: 8 in]
            n432 = local read "Internal Line Interval"() -> (w561:dbl)
            n433 = call <userlib>:"tm_setparameter_a.vi"("error in (no error)"=w571, "Value in"=w561, "Parameter"=w558, "Handle in"=w576) -> ("error out"=w565:errorcluster, "Handle out"=w567:u32)  [unwired: 6 in]
            n434 = call <userlib>:"tm_getparameter_a.vi"("error in (no error)"=w565, "Parameter"=w558, "Handle in"=w567) -> ("error out"=w564:errorcluster, "Value out"=w563:dbl, "Handle out"=w566:u32)  [unwired: 6 in]
            n435 = local write "Internal Line Interval"(w563) -> ()
            n436 = call <userlib>:"tm_preparecapture.vi"("error in (no error)"=w564, "Capture mode"=w569, "Handle in"=w566) -> ("error out"=w572:errorcluster, "Buffer Info"=w562:T7, "Handle out"=w575:u32)  [unwired: 5 in, 1 out]
            n437 = call <userlib>:"tm_startcapture_b.vi"("error in (no error)"=w572, "Handle in"=w575) -> ("error out"=w573:errorcluster, "Handle out"=w574:u32)  [unwired: 8 in]
          }
          frame "Disengage Update" {
          }
        }
        n438 = local read "stop"() -> (w158:bool)
        n439 = Compound Arithmetic op=OR(w158, w157) -> (w156:bool)
      }
      n440 = call <userlib>:"tm_stopcapture.vi"("error in (no error)"=w24, "Handle in"=w25) -> ("error out"=w71:errorcluster, "Handle out"=w72:u32)  [unwired: 8 in]
      n441 = call <userlib>:"tm_unpreparecapture.vi"("error in (no error)"=w71, "Handle in"=w72) -> ("error out"=w70:errorcluster, "Handle out"=w73:u32)  [unwired: 8 in]
      n442 = call <userlib>:"tm_closecamera.vi"("error in (no error)"=w70, "Handle in"=w73) -> ("error out"=w98:errorcluster)  [unwired: 9 in]
      n443 = call <userlib>:"tm_deinitialize.vi"("error in (no error)"=w98) -> ("error out"=w20:errorcluster)  [unwired: 10 in]
      n444 = Release Queue(queue=w19, error in (no error)=w20) -> (error out=w18:errorcluster)  [unwired: 1 in, 2 out]
      n445 = Release Queue(queue=w16, error in (no error)=w18) -> (error out=w17:errorcluster)  [unwired: 1 in, 2 out]
    }
  }
  "error out" <- w4
